vi "Text control 2 v6.3.vi"() -> ()   [LabVIEW 2016]
panel:
  in  "Tab Control":enum32{"Main", "Other parameters"}(tab)
  out "Line running":i32
  out "Total lines":i32
  out "Path":path=path "C:/users/rlp38/09Apr2009LTtesting/test2.txt"
  out "I vs Vg":cluster{"Y data in":dbl[], "X data in":dbl[]}[](graph)
  out "Is max":dbl format="%.2e"
  out "Id max":dbl format="%.2e"
  out "Ig max":dbl format="%.2e"
  out "Imax vs time":cluster{"Y data in":dbl[], "X data in":dbl[]}[](graph)
  out "Imin vs time":cluster{"Y data in":dbl[], "X data in":dbl[]}[](graph)
  out "I vs Vd":cluster{"Y data in":dbl[], "X data in":dbl[]}[](graph)
  in  "Script":string="#pulsedstressV d 0.03 20 0 0.5 0.0827 5\n#\n#itime m\n#gaterangemode a\n#drainrangemode a\n#pulsed on 0.05 0 0.02\n#transfer d -10 40 1 5 40 35\n#transfer d -10 40 1 5 40 35\n#transfer d -10 40 1 5 40 35\n#output d 0 40 20 0 40 1\n#\n#\n#sample 1 0.008 221 6 0.003\n#samplei 400e-6 200 6 0.002 0.1\n#vsu2pulse -10 4\n#\n#stressV 0.016 0.03 2e-4 0.1e-3 11\n#stressI 220e-7 0.08 15\n#transfer s -1 1 0.5 -0.005 0.005 0.005\n#output s 0 0 0 -0.008 0.008 0.002"
  out "Command running:":string
  out "Serial port data":string
  out "Elapsed Time":dbl caption="Elapsed Time (s)"
  in  "Time Units":u16(ring)=1 items=["Seconds", "Minutes", "Hours"]
  in  "Time Offset":dbl caption="Set Start Time (s)"
  in  "Reset":bool
  in  "Auto Reset":bool
  in  "integration time":u32(slide) max=2 step=1 scale=0.0..2.0
  out "Is on":dbl format="%.2e"
  out "Id on":dbl format="%.2e"
  out "Ig on":dbl format="%.2e"
  out "Ion vs time":cluster{"Y data in":dbl[], "X data in":dbl[]}[](graph)
  out "Ioff vs time":cluster{"Y data in":dbl[], "X data in":dbl[]}[](graph)
  out "Ig min":dbl format="%.2e"
  out "Id min":dbl format="%.2e"
  out "Is min":dbl format="%.2e"
  out "Is off":dbl format="%.2e"
  out "Id off":dbl format="%.2e"
  out "Ig off":dbl format="%.2e"
  in  "Integration time (long)":dbl=0.32 min=0.04 max=2.0 step=0.02 format="%.2f"
  in  "Integration time (short)":dbl=0.0019 min=8e-05 max=0.0019 step=8e-05 format="%^.0e"
  in  "Drain: Compliance":dbl=0.001 format="%.8f"
  in  "Gate: Compliance":dbl=0.001 format="%.8f"
  in  "Interrupt scan":bool
  in  "Standby":T1
  in  "Full Reset":bool
  in  "SMU4":cluster{"on/off":bool, "Voltage":dbl} {"Voltage" min=-100.0 max=100.0 format="%.2f"}
  in  "Interrupt program":bool
  in  "Gate Range\nmode":u16(ring) items=["Auto", "Limited", "Fixed"]
  in  "Gate Range":u8(slide)=6 max=11 scale=0.0..11.0
  in  "Source/Drain\nRange mode":u16(ring) items=["Auto", "Limited", "Fixed"]
  in  "Source/Drain Range":u8(slide)=6 max=11 scale=0.0..11.0
  in  "Panel Controls":T2={"Emergency Stop"=refnum, "TransGraph Max"=1e-05, "Text/Graph (text=false)"=TRUE} {"TransGraph Max" format="%.2e"}
  in  "Panel Controls 2":T3={"Emergency Stop"=refnum, "TransGraph Max"=1e-05, "Text/Graph (text=false)"=TRUE, "TransGraph Min"=1e-11} {"TransGraph Min" format="%.2e"; "TransGraph Max" format="%.2e"}
  out "error out":errorcluster
  in  "Delay before read (ms)":u32=1000
  in  "byte count":u32=64
  in  "Serial End Mode for Reads":u16(ring)=2 items=["None", "LastBit", "TermChar"]
  in  "Timeout (ms)":u32=10000
  in  "Enable Termination\nChar (T)":bool=TRUE
  in  "Termination char\n(0xA = '\\n' = LF)\n(0xD = '\\r' = CR)":u8=13 format="%.0x"
  in  "flow control":u16(ring) items=["None"=0, "XON/XOFF"=1, "RTS/CTS"=2, "DTR/DSR"=4]
  in  "stop bits":u16(ring)=10 items=["1.0"=10, "1.5"=15, "2.0"=20]
  in  "parity":u16(ring) items=["None", "Odd", "Even", "Mark", "Space"]
  in  "data bits":u16=8 min=5 max=8 step=1
  in  "VISA resource name":refnum<visa-resource-name>="COM6"
  in  "baud rate":u32=9600
  out "Timings Indicator":T4
  in  "Timings (overwritten by the Front Panel)":T5={"integration time"=0, "Short/Long integration time"=0.00064, "hold time (sec)"=0.0, "delay time (sec)"=0.0, "Step Time (0 disables)"=0.0, "sweep method"=0, "Pulse period"=0.005, "Base voltage"=0.0, "Pulse width"=0.0005} {"Pulse width" min=0.0005 max=0.1 step=0.0001 format="%.4f"; "Base voltage" format="%^.4e"; "Pulse period" min=0.005 max=1.0 step=0.0001 format="%.4f"; "sweep method" items=["Continuous", "Pulsed"]; "Step Time (0 disables)" format="%.2f"; "delay time (sec)" format="%.4f"; "hold time (sec)" format="%.4f"; "Short/Long integration time" format="%^.0e"; "integration time" scale=0.0..2.0}
  in  "Gate":T6={"Gate Start"=0.0, "Gate Stop"=2.0, "Gate Step (linear only)"=1.0, "Gate Compliance"=0.0001, "Gate PComp"=0.0, "Range mode"=0, "Range"=6} {"Range" max=11 scale=0.0..11.0; "Range mode" items=["Auto", "Limited", "Fixed"]; "Gate PComp" format="%^.2e"; "Gate Compliance" format="%^.2e"; "Gate Step (linear only)" format="%^.4e"; "Gate Stop" format="%^.4e"; "Gate Start" format="%^.4e"}
  in  "Drain 2":T7={"Drain Start"=0.0, "Drain Stop"=2.0, "Drain Compliance"=0.0001, "Drain Step"=1.0, "Drain PComp"=0.0, "Range mode"=0, "Range"=6} {"Range" max=11 scale=0.0..11.0; "Range mode" items=["Auto", "Limited", "Fixed"]; "Drain PComp" format="%^.2e"; "Drain Step" format="%^.4e"; "Drain Compliance" format="%^.2e"; "Drain Stop" format="%^.4e"; "Drain Start" format="%^.4e"}
  # "Time"
  # "Syntax:\nitime [s|m|l] time(sec): [s|m|l] determines the integration time setting (small|medium|long) and time sets the value.\nNOTE: The value of the integration time has to be within the range allowed by its category (s|m|l), otherwise, the closest value will be used. (e.g. if the category is set to short but the time value is very long, the actual value used will be the maximum short integration time.\nIntegration times:\n    Short: Default: 640 us. Range: 8E-5 - 1.92E-3 seconds.\n    Medium: Fixed at 1 NPL cycle (0.02 seconds).\n    Long: Default: 16 NPL cycles (0.32 seconds). Range: 2-100 NPL cycles (0.04 seconds - 2 seconds).\ngaterangemode [a|l|f]\ndrainrangemode [a|l|f]\npulsed [on|off] PulsePeriod(sec) PulseBaseVoltage PulseONWidth(sec)\nstandby [on l off]\nwait NumMilliseconds\nwait-min NumMinutes\n# texthere = comment\ntransfer [s|d] VgStart VgStop VgStep VdStart VdStop VdStep\noutput [s|d] VgStart VgStop VgStep VdStart VdStop VdStep\nsample Vg Vd NumSamples Time(s) SampleInterval(s)\nsamplei Idg NumSamples Time(s) SampleInterval(s) VDGcompliance\n100 samples is approximately 13 seconds with medium integration\n# if in doubt use SampleInterval(s) = 0.004\nstressV VG VD IGcompliance IDcompliance Duration(sec)\nstressI IDG VDGcompliance Duration(sec)\nvsu2pulse Bias Duration(s)\npulsedstressV [s|d] VEstop VgON VgOFF Period(s) PulseONwidth(s) Vd\nsample-fpp Vg Vd NumSamples Time\nresample-fpp Vg Vd\ntransfer-fpp [s|d] VgStart VgStop VgStep VdStart VdStop VdStep\noutput-fpp [s|d] VgStart VgStop VgStep VdStart VdStop VdStep\nserial SerialPortCommand"
  # "1\n2\n3\n4\n5\n6\n7\n8\n9\n10\n11\n12\n13\n14\n15\n16\n17\n18\n19\n20"
  # "Serial port settings"
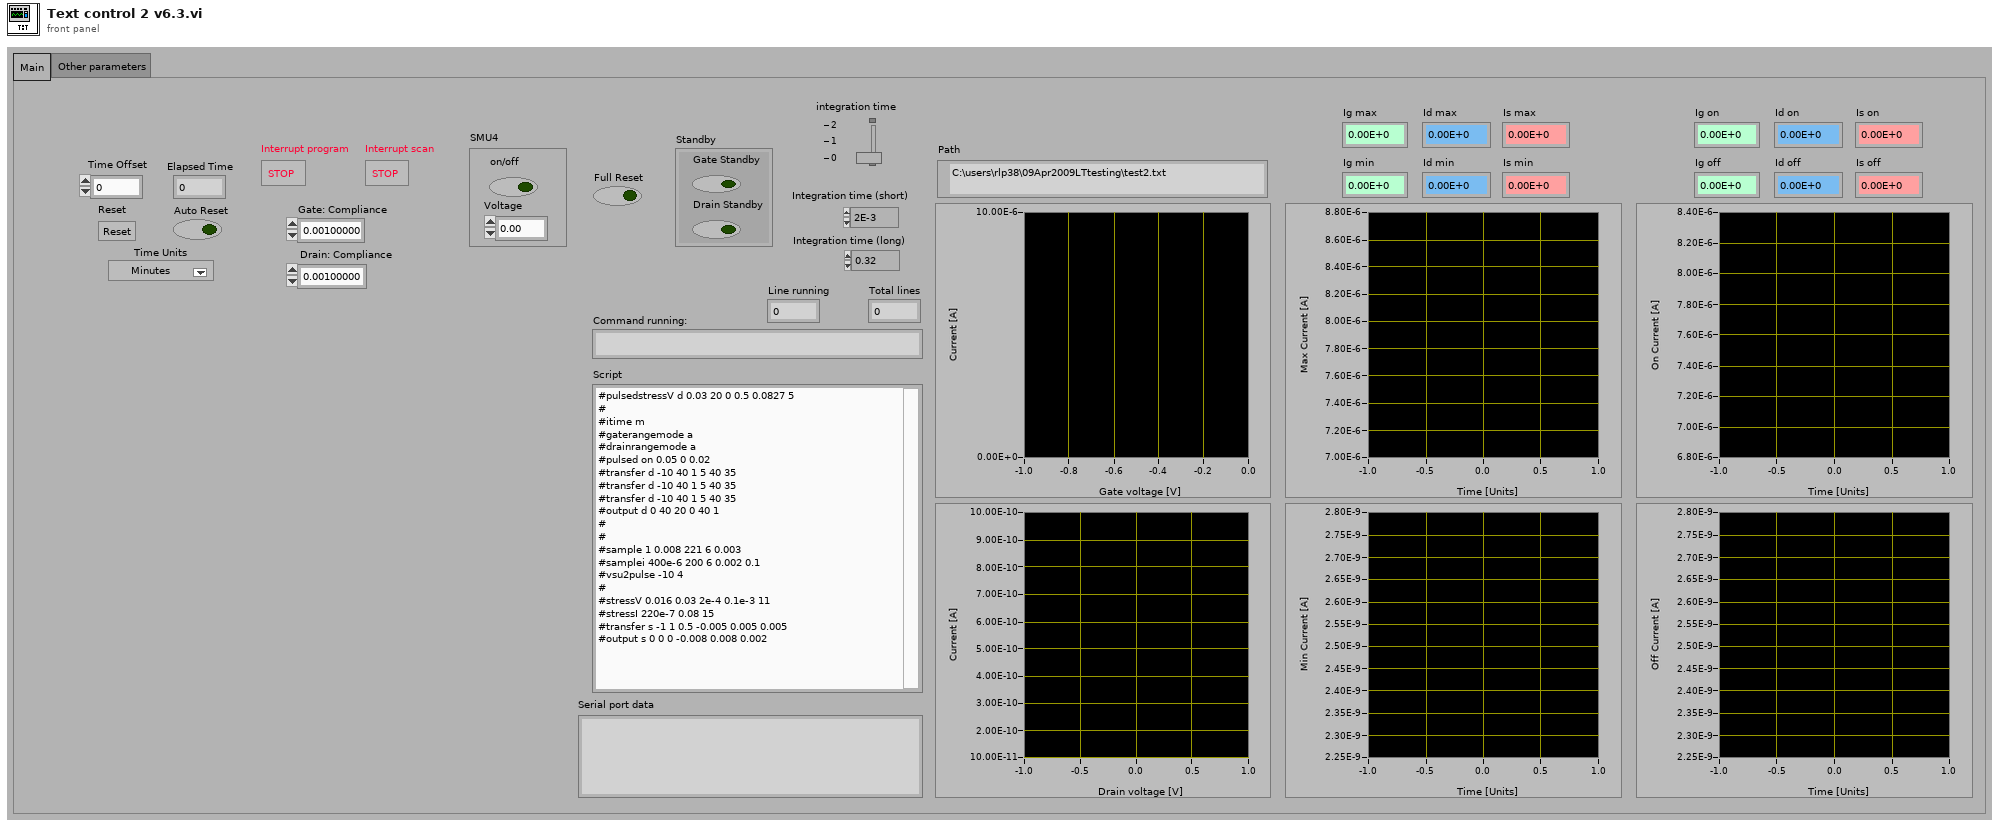
[diagram p1: front panel]
types:
  T1 = cluster{"Gate Standby":bool, "Drain Standby":bool}
  T2 = cluster{"Emergency Stop":refnum<vi>, "TransGraph Max":dbl, "Text/Graph (text=false)":bool}
  T3 = cluster{"Emergency Stop":refnum<vi>, "TransGraph Max":dbl, "Text/Graph (text=false)":bool, "TransGraph Min":dbl}
  T4 = cluster{"integration time (0:s, 1:m, 2:l)":u32, "Short/Long integration time":dbl, "hold time (sec)":dbl, "delay time (sec)":dbl, "Step Time (0 disables)":dbl, "sweep method":u16, "Pulse period":dbl, "Base voltage":dbl, "Pulse width":dbl}
  T5 = cluster{"integration time":u32, "Short/Long integration time":dbl, "hold time (sec)":dbl, "delay time (sec)":dbl, "Step Time (0 disables)":dbl, "sweep method":u16, "Pulse period":dbl, "Base voltage":dbl, "Pulse width":dbl}
  T6 = cluster{"Gate Start":dbl, "Gate Stop":dbl, "Gate Step (linear only)":dbl, "Gate Compliance":dbl, "Gate PComp":dbl, "Range mode":u16, "Range":u8}
  T7 = cluster{"Drain Start":dbl, "Drain Stop":dbl, "Drain Compliance":dbl, "Drain Step":dbl, "Drain PComp":dbl, "Range mode":u16, "Range":u8}
  T8 = enum16{"open", "replace", "create", "open or create", "replace or create", "replace or create with confirmation"}
  T9 = cluster{"V2 Start":dbl, "V2 Step":dbl, "Number of points":i32}
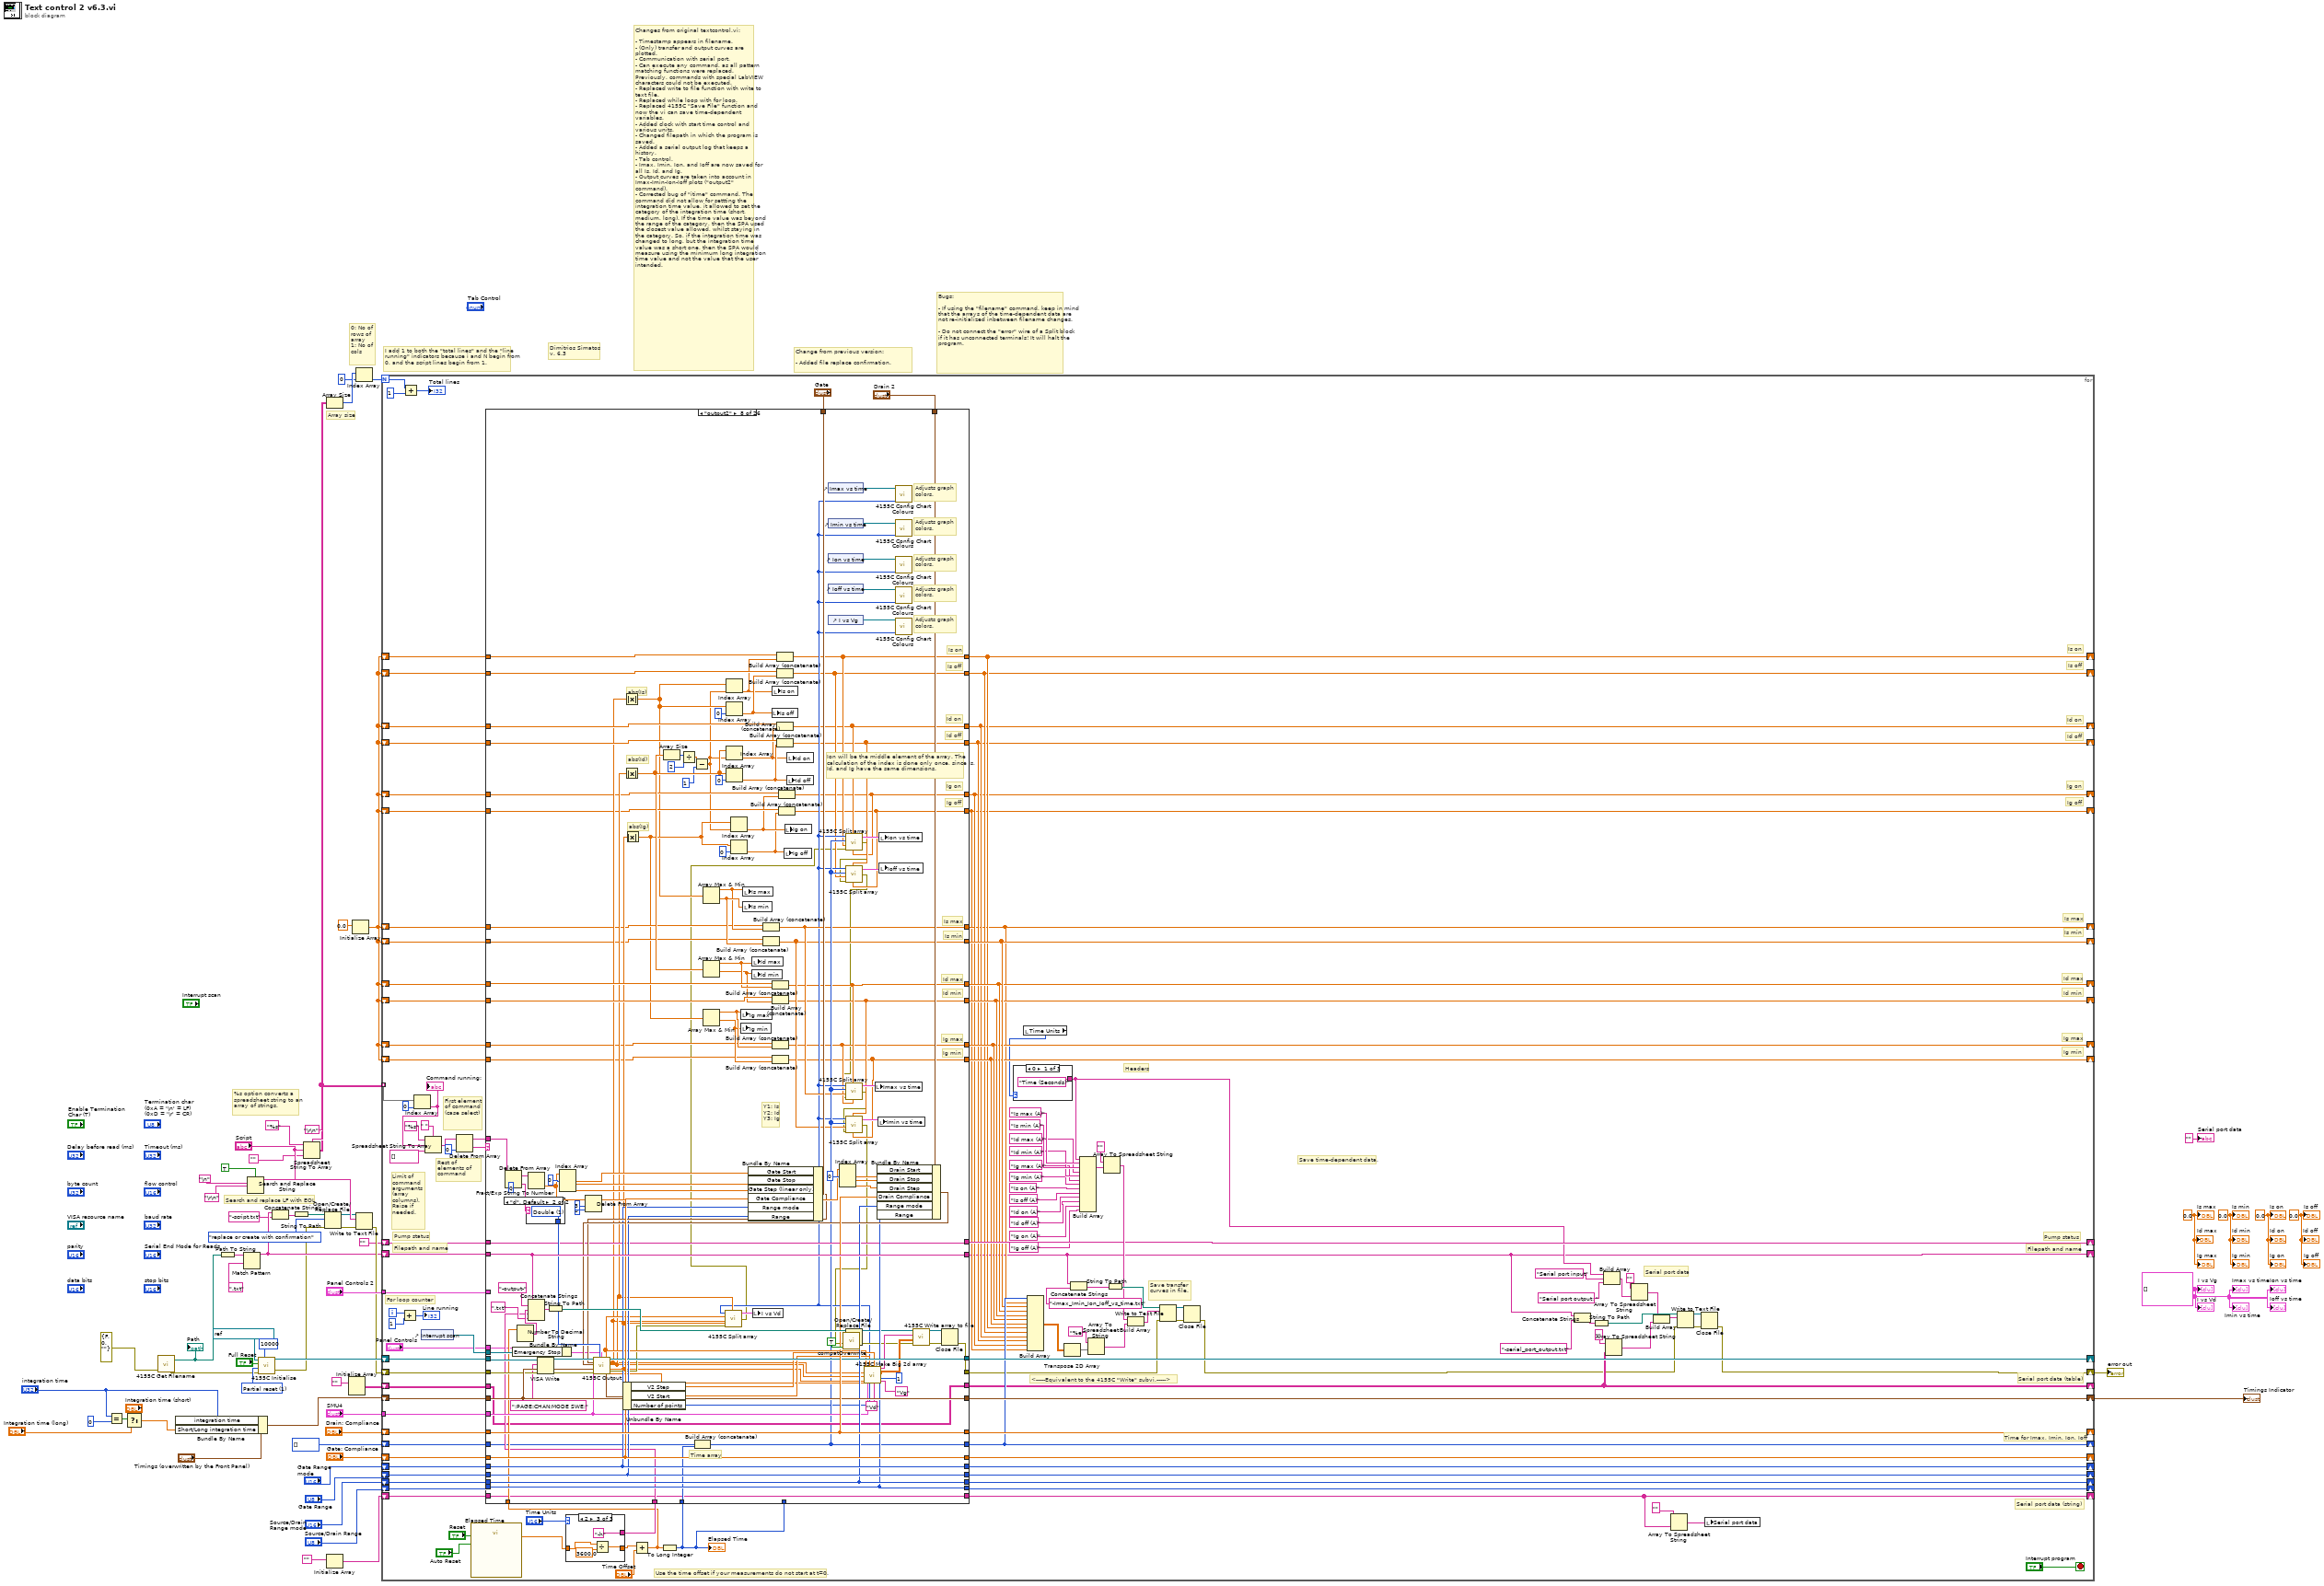
[diagram p0: block diagram]
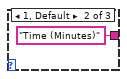
[diagram p2: hidden frame]
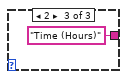
[diagram p3: hidden frame]
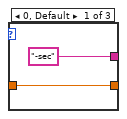
[diagram p4: hidden frame]
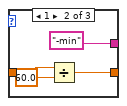
[diagram p5: hidden frame]
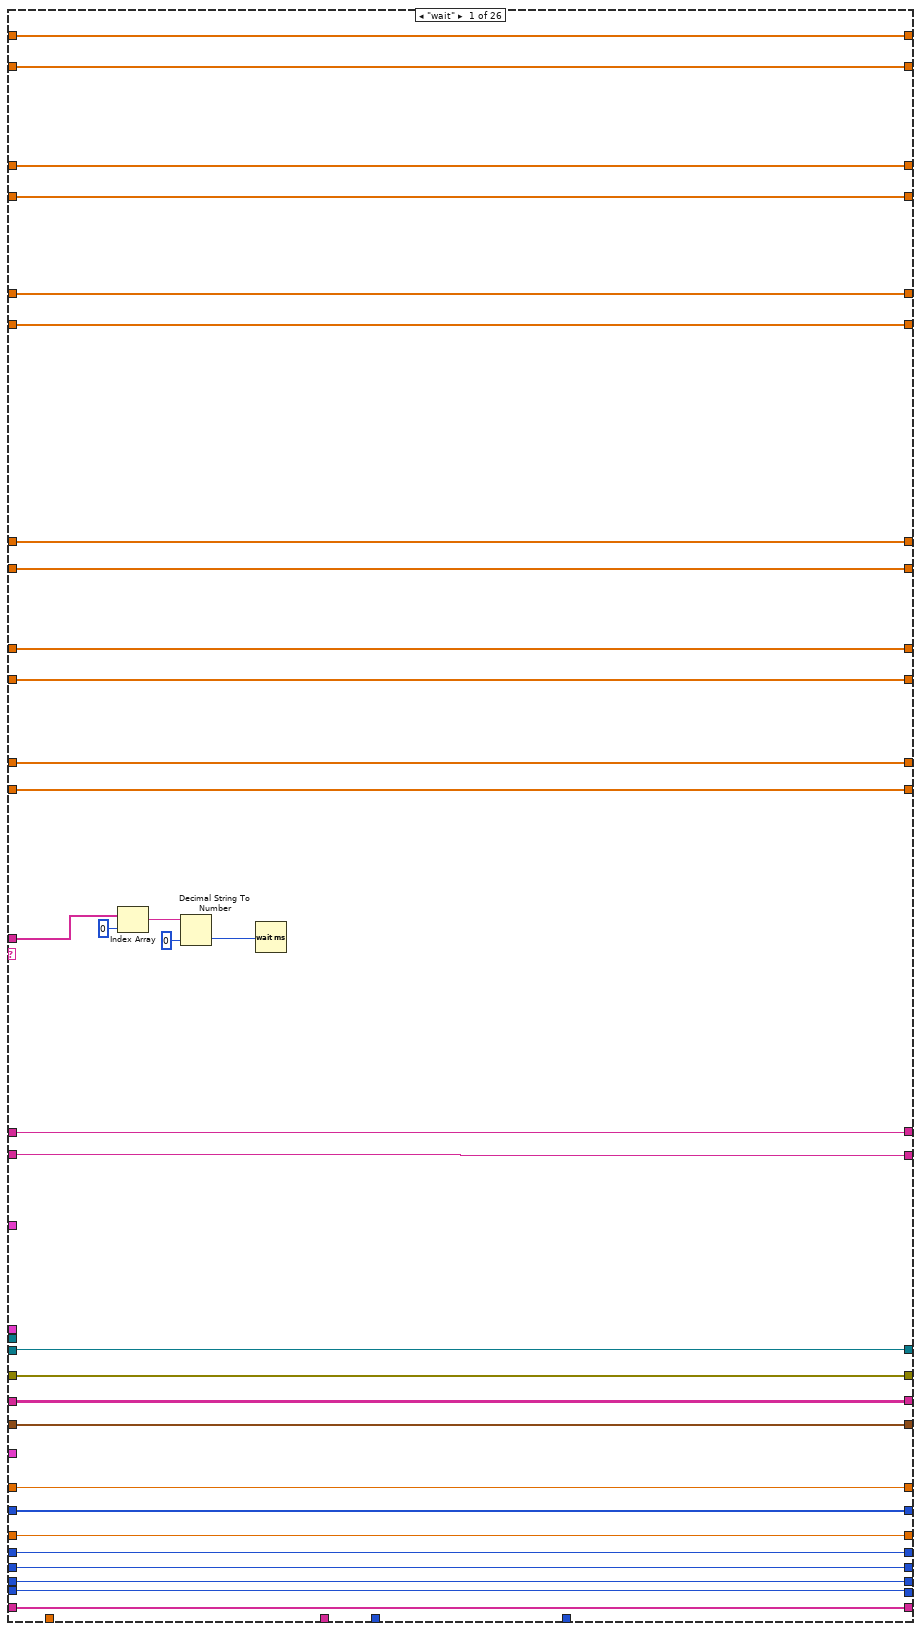
[diagram p6: hidden frame]
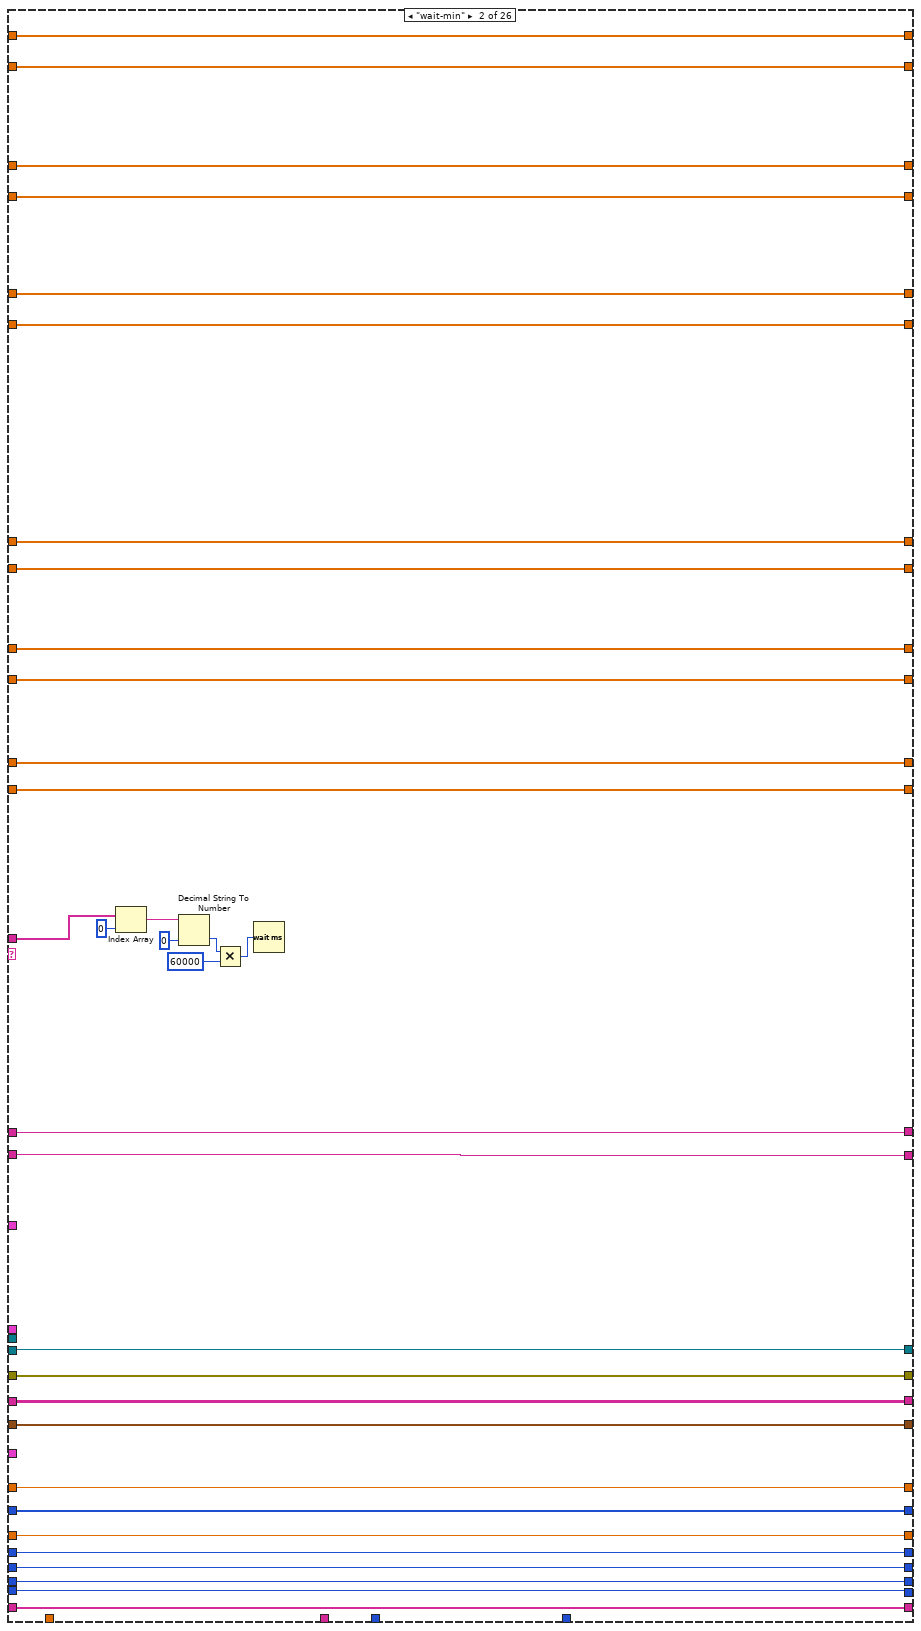
[diagram p7: hidden frame]
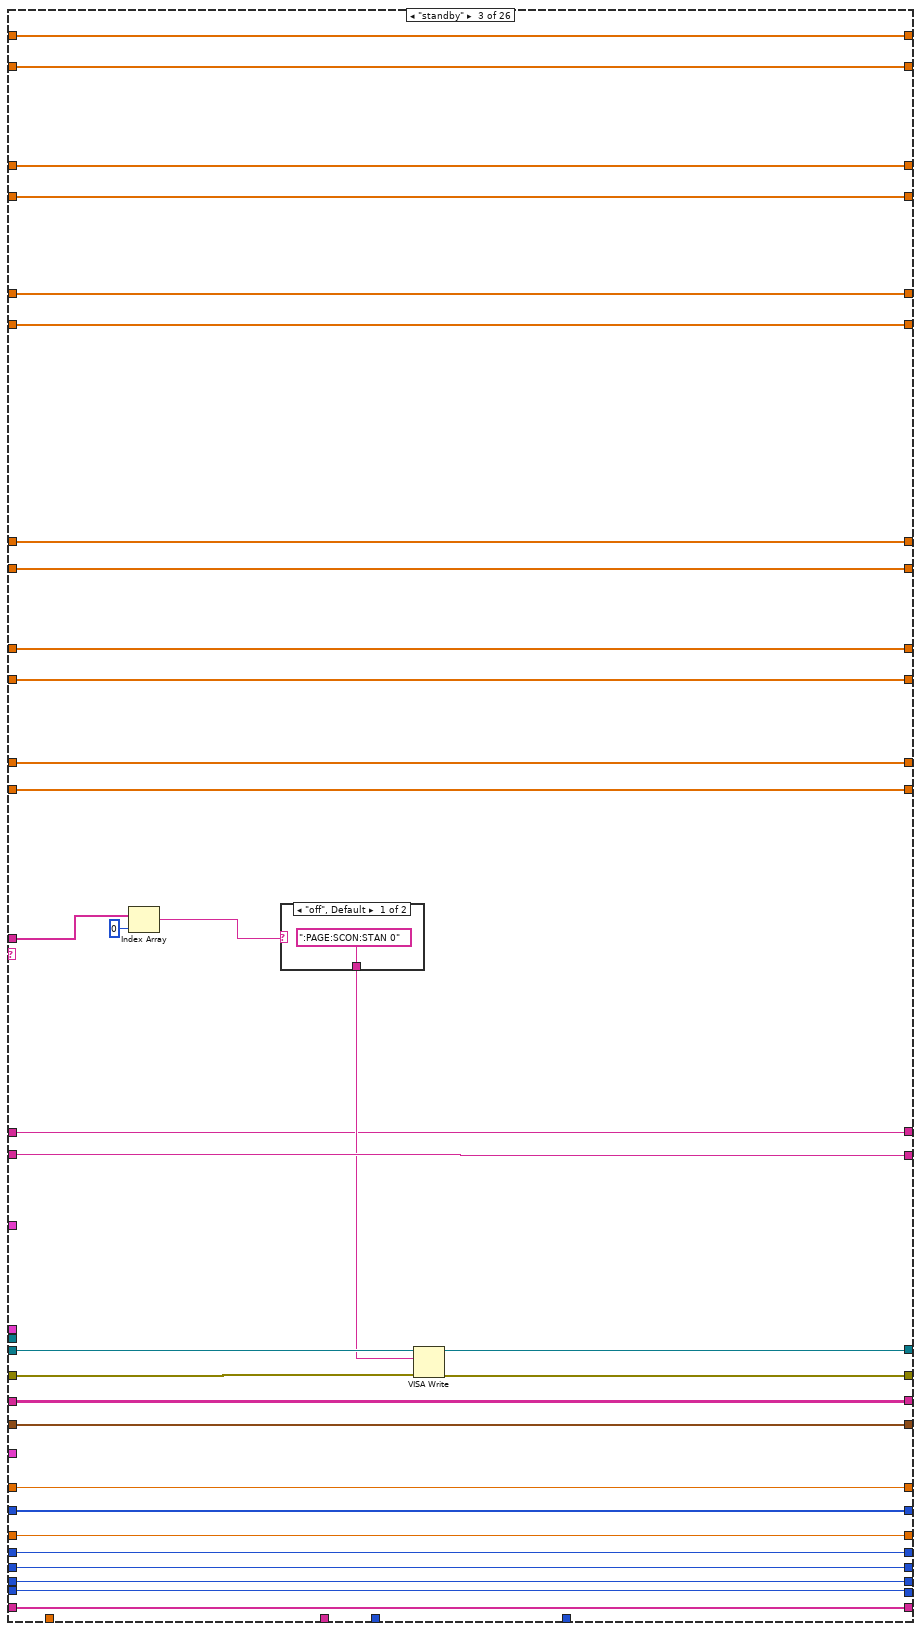
[diagram p8: hidden frame]
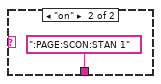
[diagram p9: hidden frame]
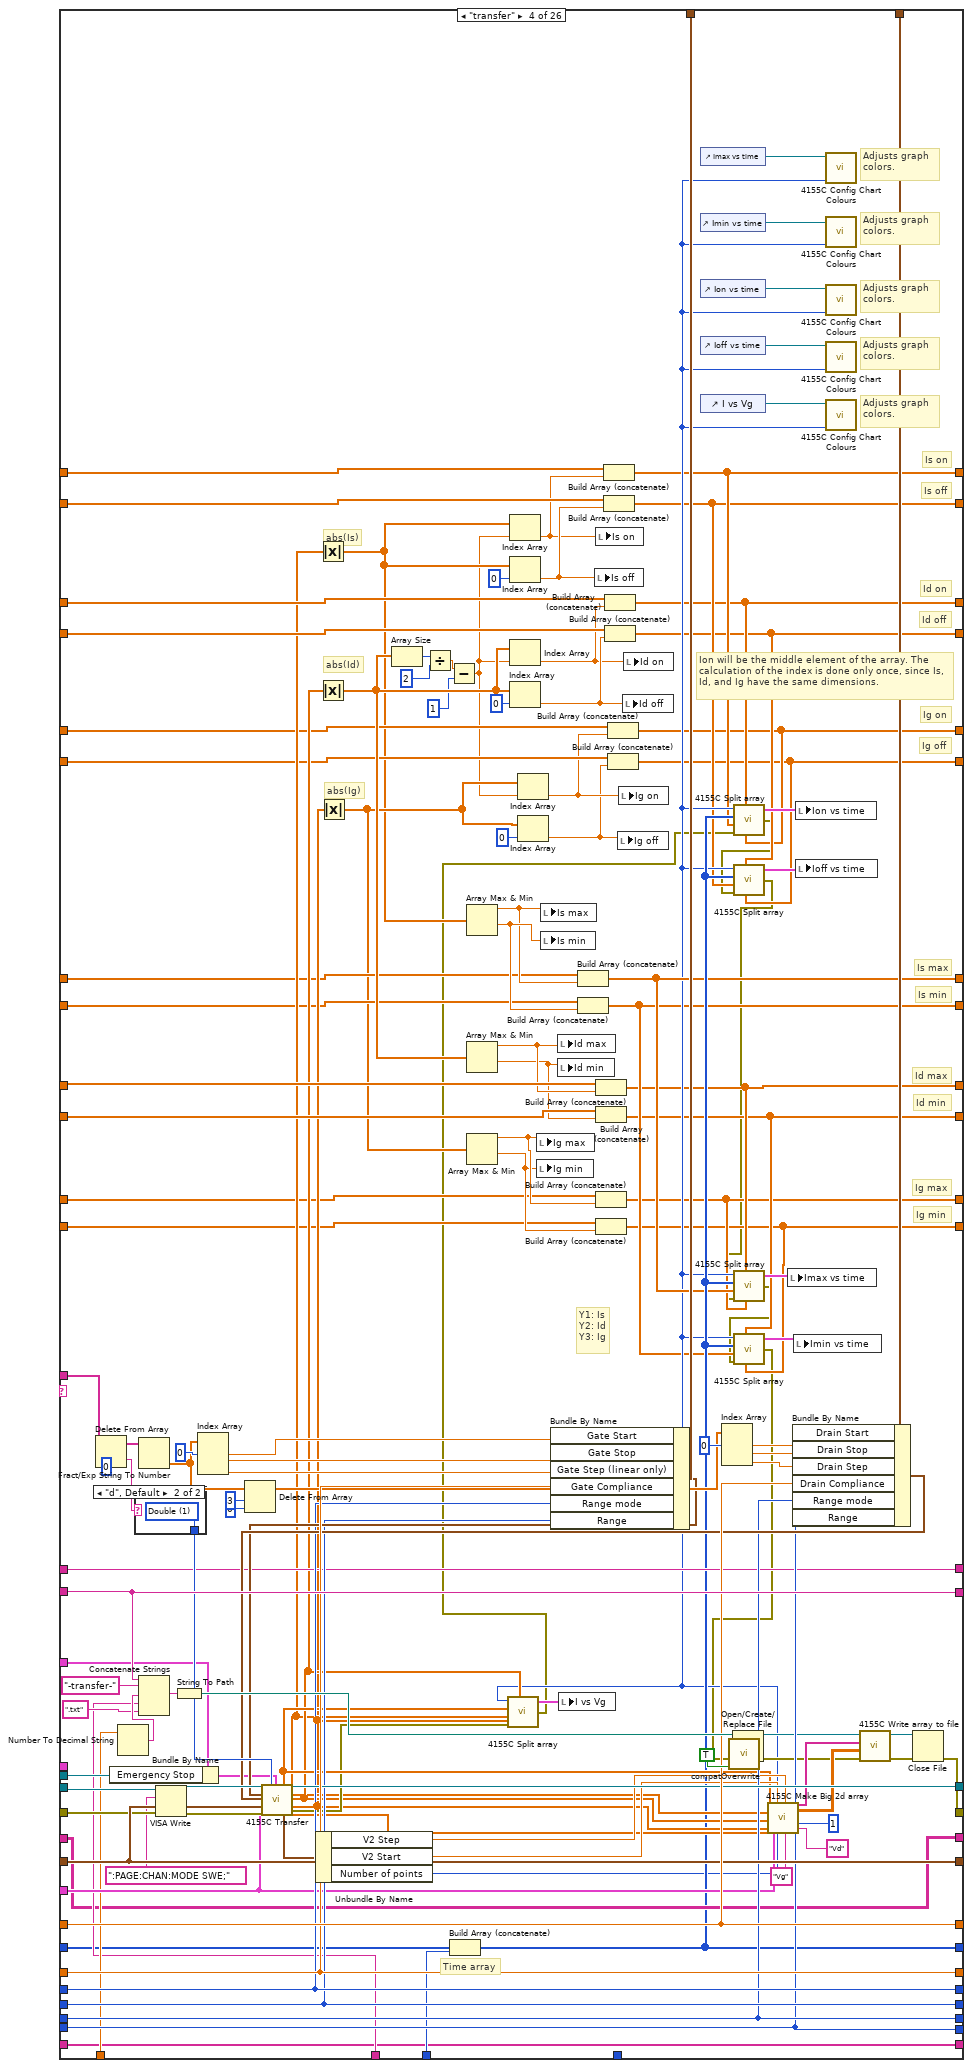
[diagram p10: hidden frame]
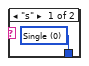
[diagram p11: hidden frame]
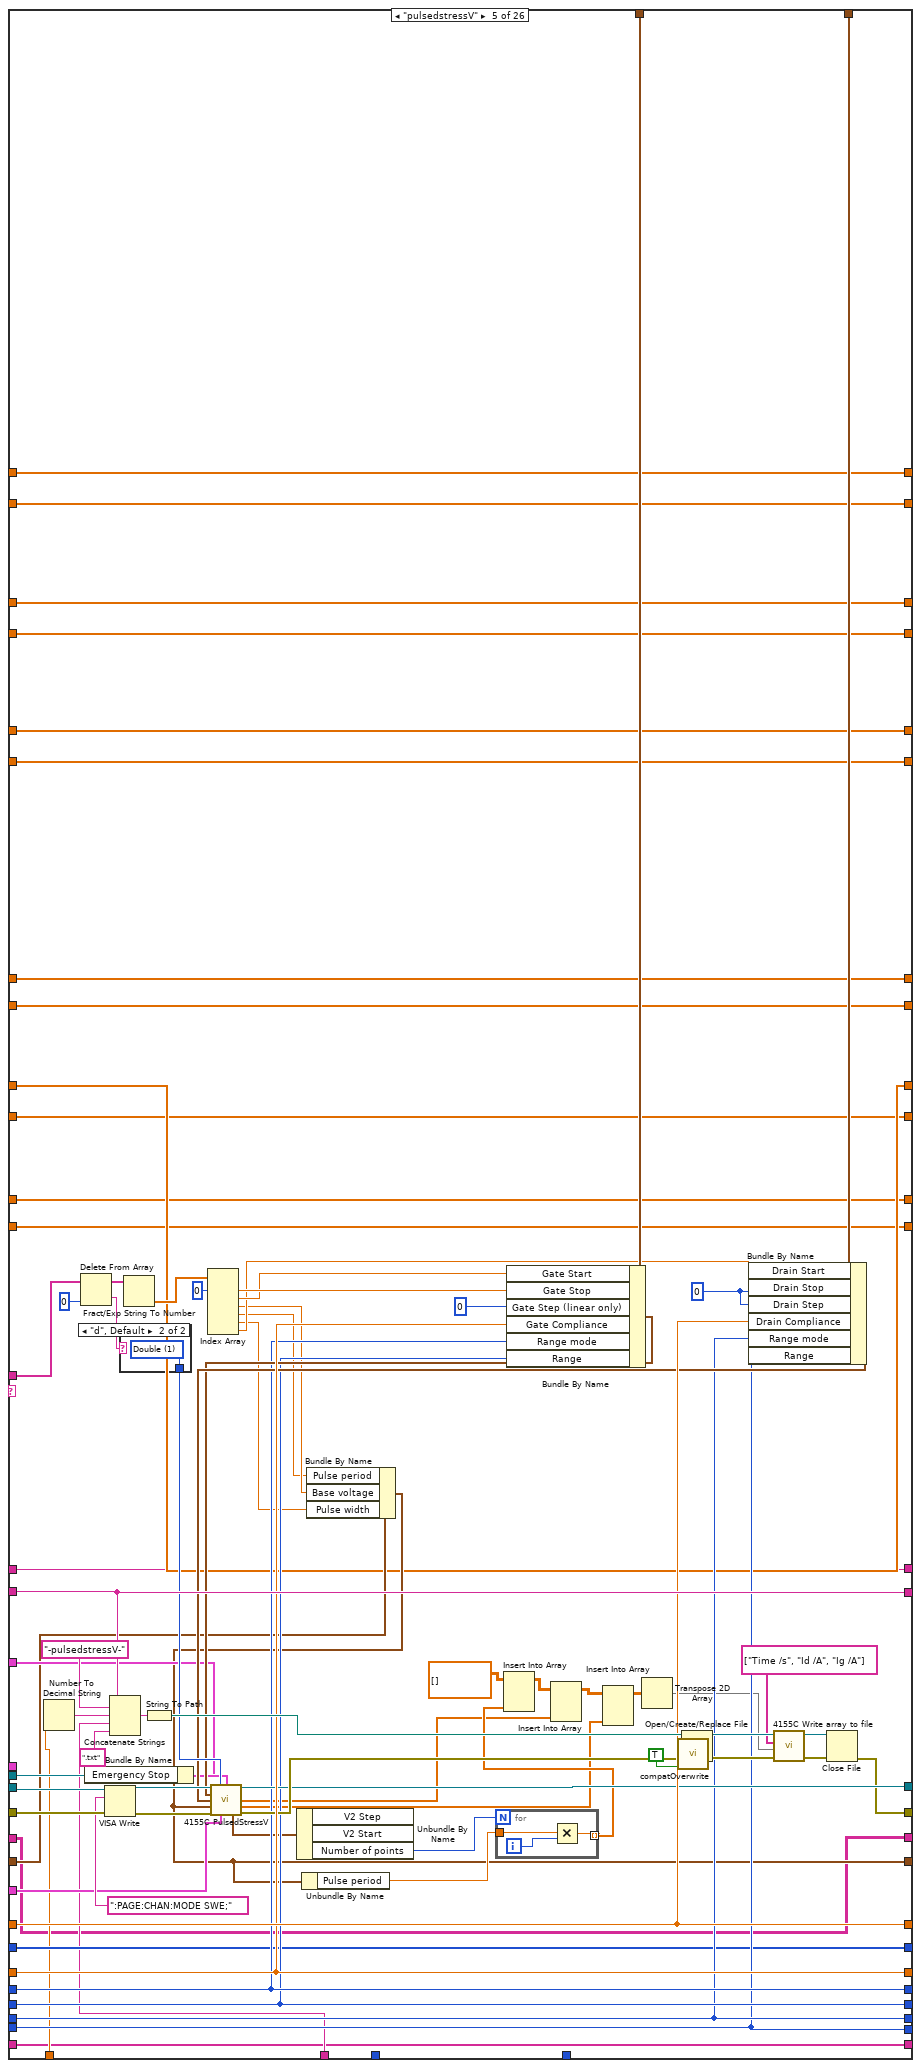
[diagram p12: hidden frame]
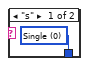
[diagram p13: hidden frame]
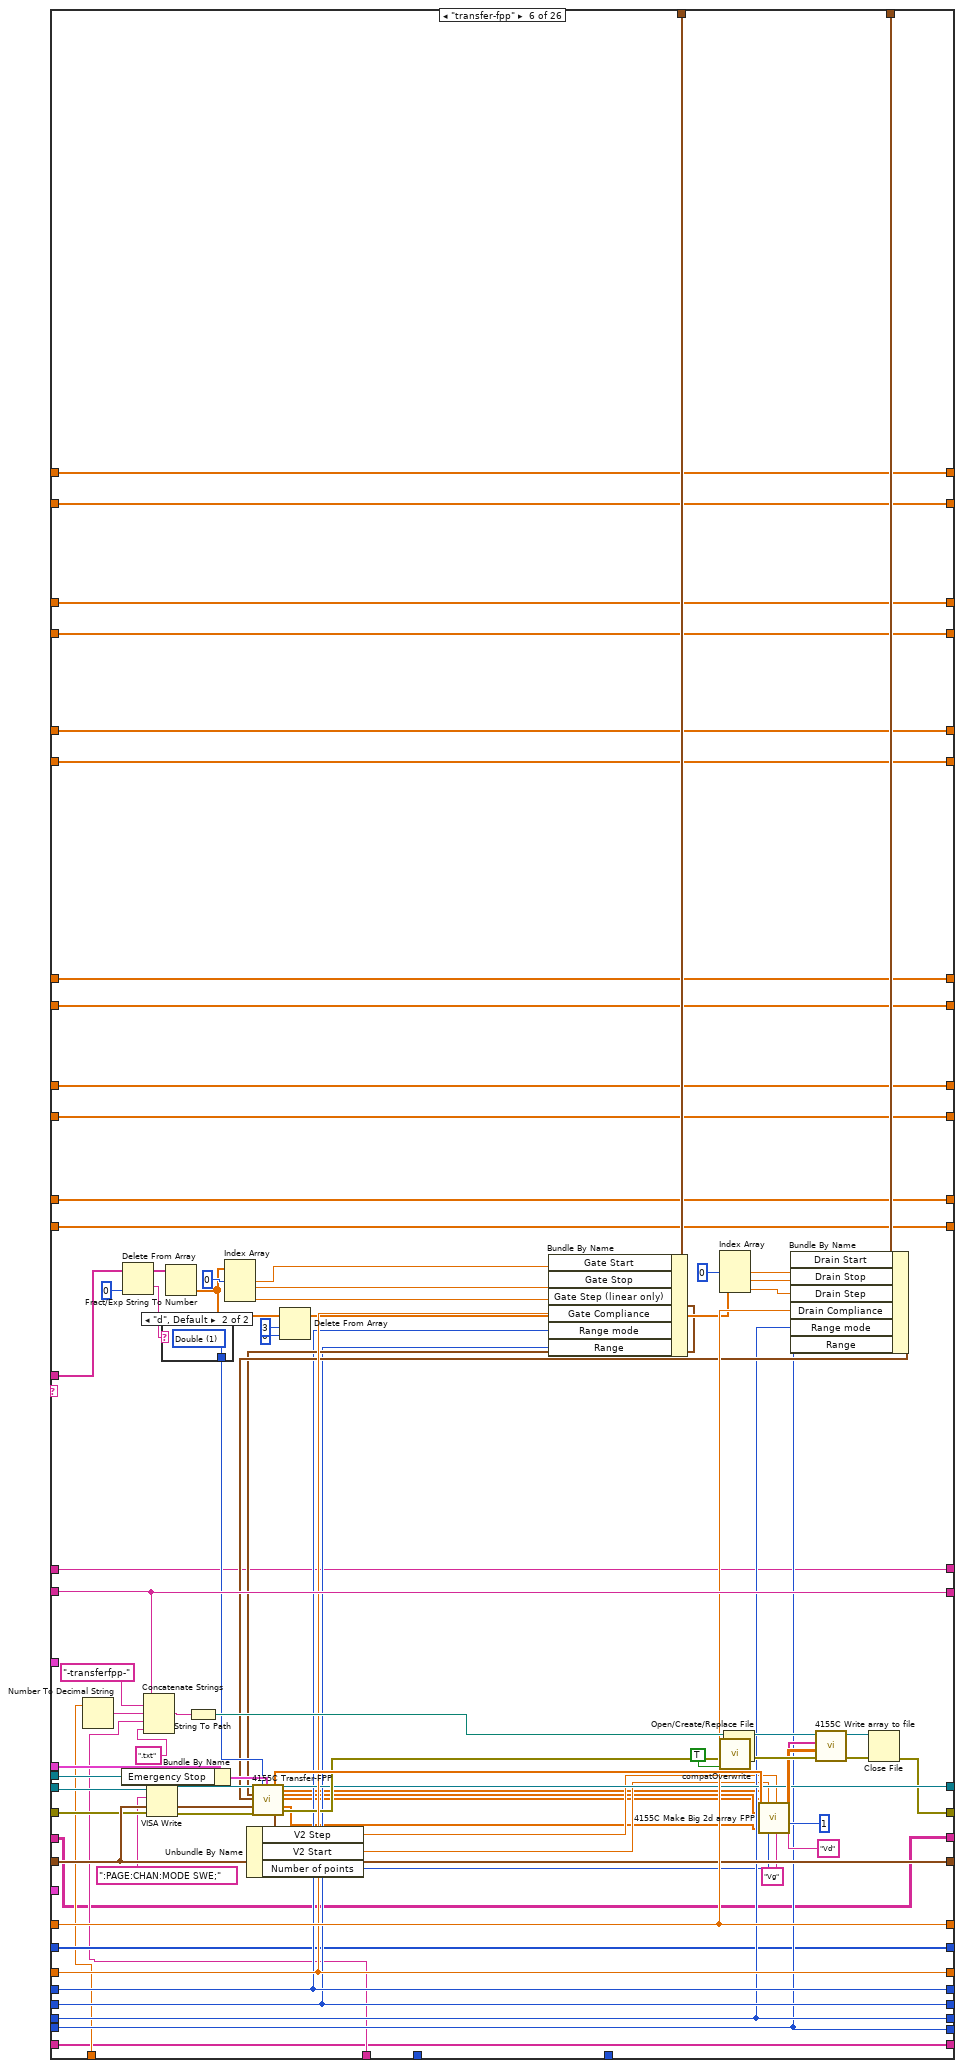
[diagram p14: hidden frame]
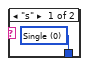
[diagram p15: hidden frame]
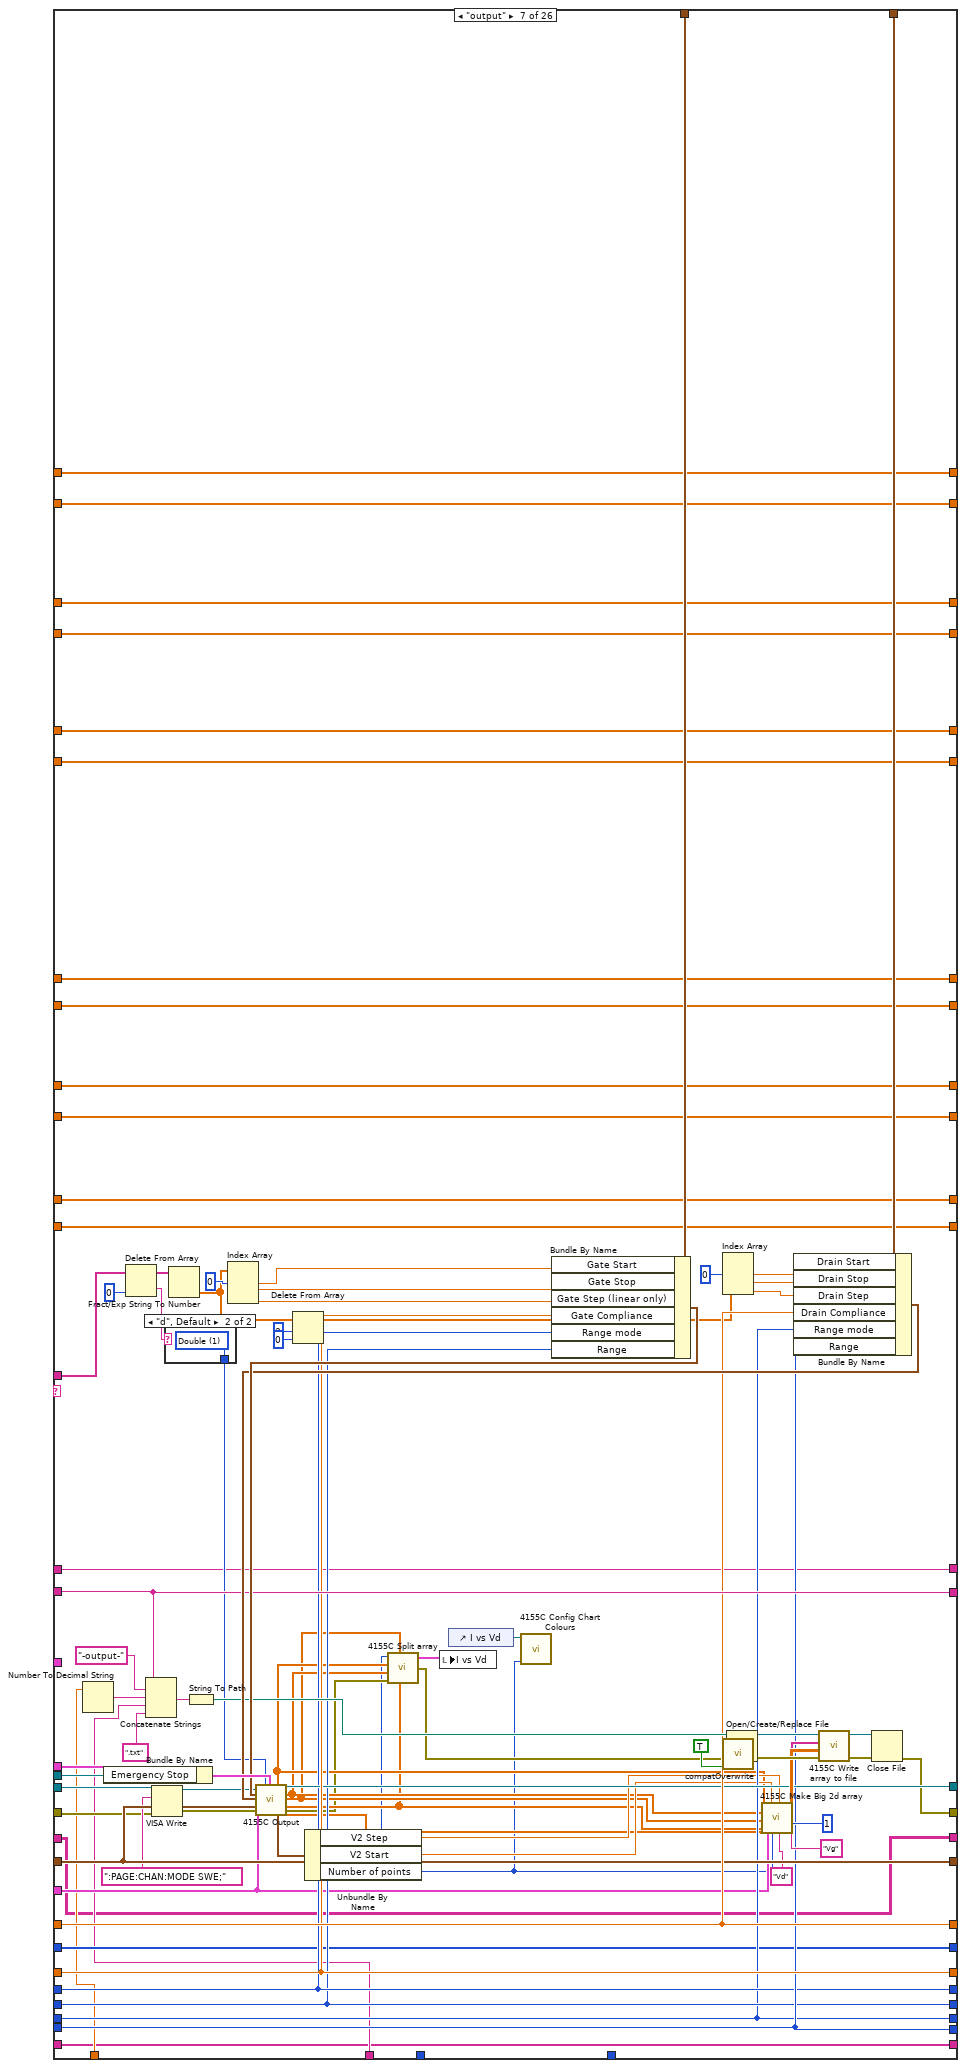
[diagram p16: hidden frame]
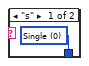
[diagram p17: hidden frame]
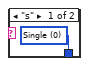
[diagram p18: hidden frame]
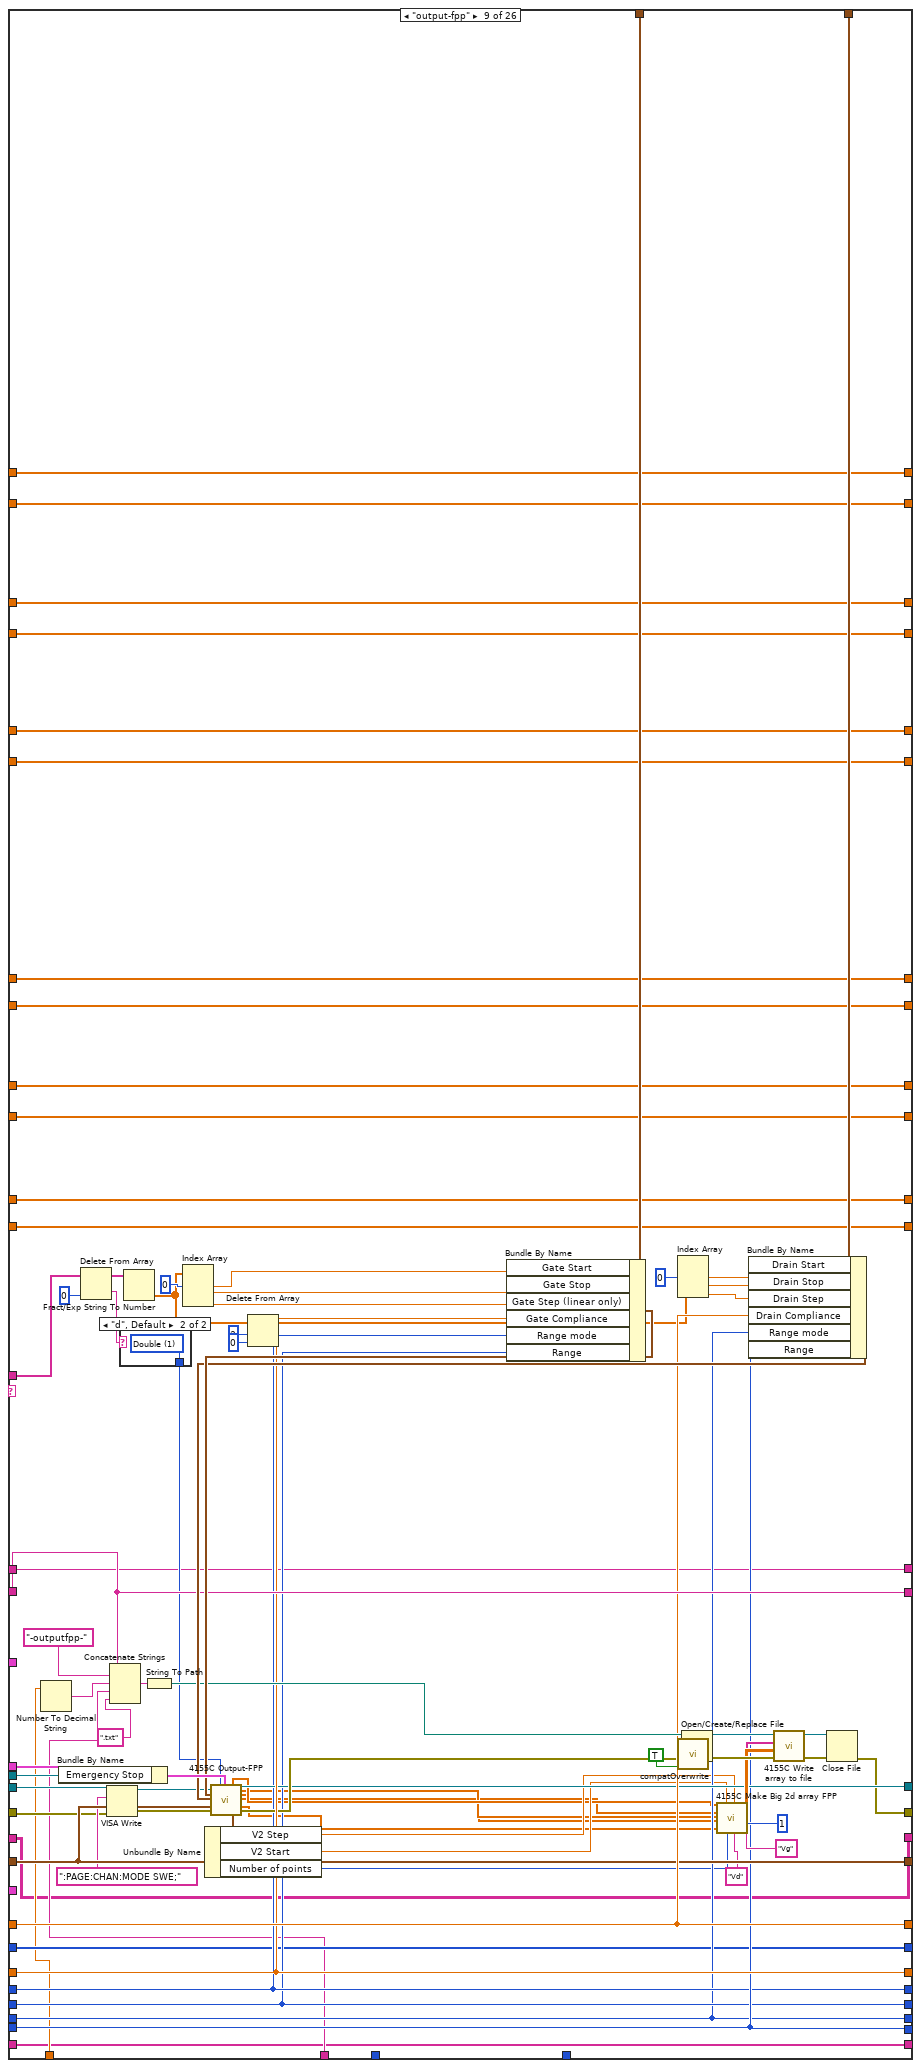
[diagram p19: hidden frame]
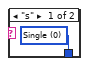
[diagram p20: hidden frame]
diagram:
  w7 = cluster{"Y data in":dbl[], "X data in":dbl[]}[] [] ("I vs Vg")
  w8 = 0.0 ("Is off")
  w9 = 0.0 ("Is on")
  w10 = 0.0 ("Is min")
  w11 = 0.0 ("Is max")
  w58 = u16 1 items=["Reset All", "Partial reset"] ("Type of reset")
  # "Change from previous version:\n\n- Added file replace confirmation."
  # "I add 1 to both the \"total lines\" and the \"line running\" indicators because i and N begin from 0, and the script lines begin from 1."
  # "Bugs:\n\n- If using the \"filename\" command, keep in mind that the arrays of the time-dependent data are not re-initialized inbetween filename changes. \n\n- Do not connect the \"error\" wire of a Split block if it has unconnected terminals! It will halt the program."
  # "Array size"
  # "%s option converts a spreadsheet string to an array of strings."
  # "0: No of rows of array\n1: No of cols"
  # "Dimitrios Simatos\nv. 6.3"
  # "Changes from original textcontrol.vi:\n\n- Timestamp appears in filename.\n- (Only) transfer and output curves are plotted.\n- Communication with serial port.\n- Can execute any command, as all pattern matching functions were replaced. Previously, commands with special LabVIEW characters could not be executed.\n- Replaced write to file function with write to text file.\n- Replaced while loop with for loop.\n- Replaced 4155C \"Save File\" function and now the vi can save time-dependent variables.\n- Added clock with start time control and various units.\n- Changed filepath in which the program is saved.\n- Added a serial output log that keeps a history.\n- Tab control.\n- Imax, Imin, Ion, and Ioff are now saved for all Is, Id, and Ig.\n- Output curves are taken into account in Imax-Imin-Ion-Ioff plots (\"output2\" command).\n- Corrected bug of \"itime\" command. The command did not allow for settting the integration time value, it allowed to set the category of the integration time (short, medium, long). If the time value was beyond the range of the category, then the SPA used the closest value allowed, whilst staying in the category. So, if the integration time was changed to long, but the integration time value was a short one, then the SPA would measure using the minimum long integration time value and not the value that the user intended."
  # "Search and replace LF with EOL"
  n1 = Equal?(x="integration time", y=u32 0) -> (x = y?=w59:bool)
  n2 = Select(t="Integration time (short)", s=w59, f="Integration time (long)") -> (s? t:f=w16:dbl)
  n3 = call "4155C Get Filename.vi"("error in (no error)"=errorcluster {"status"=FALSE, "code"=0, "source"=""}) -> ("error out"=w53:errorcluster, "path"=w28:path)  [unwired: 2 in, 1 out]
  "Path" <- w28
  n4 = Bundle By Name(cluster="Timings (overwritten by the Front Panel)", "integration time"="integration time", "Short/Long integration time"=w16) -> (w51:T5)
  n5 = Path To String(path=w28) -> (string=w29:string)
  n6 = Match Pattern(string=w29, regular expression=".txt") -> (before substring=w14:string)  [unwired: 1 in, 3 out]
  n7 = Search and Replace String(replace all?=TRUE ("replace all? (F)"), input string="Script", search string="\n", replace string="\r\n") -> (result string=w41:string)  [unwired: 4 in, 3 out]
  n8 = call "4155C Initialise.vi"("VISA resource name in"=refnum<visa-resource-name> "GPIB0::14::INSTR", "Reset"="Full Reset", "Type of reset"=w58, "error in (no error)"=w53, "VISA Timeout Value"=u32 10000) -> ("VISA Resource Name out"=w52:refnum<visa-resource-name>, "error out"=w5:errorcluster)
  n9 = Concatenate Strings(w14, "-script.txt" ("string")) -> (w15:string)
  n10 = String To Path(string=w15) -> (path=w3:path)
  n11 = Spreadsheet String To Array(delimiter (Tab)="\r\n", format string="%s", spreadsheet string="Script", array type (2D Dbl)="") -> (array=w32:string[][])
  n12 = Open/Create/Replace File(file path (use dialog)=w3, error in=w5, operation (0:open)=T8."replace or create with confirmation") -> (refnum out=w2:refnum<file>, error out=w4:errorcluster)  [unwired: 3 in, 1 out]
  n13 = Array Size(array=w32) -> (size(s)=w36:i32[])
  n14 = Initialize Array("") -> (w21:string[])  [unwired: 1 in]
  n15 = Initialize Array("") -> (w19:string[][])  [unwired: 2 in]
  n16 = Initialize Array(0.0 ("element")) -> (w23:dbl[])  [unwired: 1 in]
  n17 = Index Array(array=w36, index=0) -> (element=w34:i32)
  n18 = Write to Text File(file (use dialog)=w2, text=w41, error in=w4) -> (error out=w25:errorcluster)  [unwired: 1 in, 2 out]
  n19 = for {
    N: w34 -> [w133]
    tunnel: "SMU4" -> [w169]
    shift-left: "Source/Drain Range" -> [w174]
    shift-right: [w170] -> _
    shift-left: "Source/Drain\nRange mode" -> [w175]
    shift-right: [w171] -> _
    shift-left: "Gate Range" -> [w176]
    shift-right: [w172] -> _
    shift-left: "Gate Range\nmode" -> [w177]
    shift-right: [w173] -> _
    shift-left: "Gate: Compliance" -> [w186]
    shift-right: [w182] -> _
    shift-left: "Drain: Compliance" -> [w187]
    shift-right: [w183] -> _
    shift-left: w51 -> [w188]
    shift-right: [w184] -> w17
    shift-left: w25 -> [w189]
    shift-right: [w67] -> w27
    shift-left: w52 -> [w190]
    shift-right: [w185] -> _
    shift-left: w14 -> [w191]
    shift-right: [w70] -> _
    tunnel: "Panel Controls 2" -> [w168]
    shift-right: [w82] -> _
    shift-left: w23 -> [w167]
    shift-right: [w118] -> _
    shift-left: i32[] [] -> [w163]
    tunnel: w32 -> [w162] mode=indexing
    shift-right: [w81] -> _
    shift-left: w23 -> [w139]
    shift-right: [w112] -> _
    shift-left: w21 -> [w125]
    shift-right: [w120] -> _
    shift-left: "" -> [w119]
    shift-right: [w113] -> _
    shift-left: w19 -> [w115]
    shift-right: [w75] -> _
    shift-left: w23 -> [w103]
    shift-right: [w76] -> _
    shift-left: w23 -> [w102]
    shift-right: [w80] -> _
    shift-left: w23 -> [w91]
    shift-right: [w79] -> _
    shift-left: w23 -> [w90]
    shift-right: [w73] -> _
    shift-left: w23 -> [w89]
    shift-right: [w83] -> _
    shift-left: w23 -> [w88]
    shift-right: [w74] -> _
    shift-left: w23 -> [w87]
    shift-right: [w72] -> _
    shift-left: w23 -> [w86]
    shift-right: [w78] -> _
    shift-left: w23 -> [w85]
    shift-right: [w77] -> _
    shift-left: w23 -> [w84]
    i -> [w128]
    stop <- "Interrupt program" stop-if-true
    # "Is off"
    # "Is on"
    # "Ig off"
    # "Ig on"
    # "Is min"
    # "Is max"
    # "Ig min"
    # "Ig max"
    # "Id min"
    # "Id max"
    # "Id off"
    # "Id on"
    # "Pump status"
    # "Filepath and name"
    # "Pump status"
    # "Limit of command arguments (array columns). Raise if needed."
    # "Serial port data (string)"
    # "Serial port data (table)"
    # "Serial port data"
    # "For loop counter"
    # "<-----Equivalent to the 4155C \"Write\" subvi.----->"
    # "Headers"
    # "Save transfer curves in file."
    # "Filepath and name"
    # "Save time-dependent data."
    # "Use the time offset if your measurements do not start at t=0."
    # "Time for Imax, Imin, Ion, Ioff"
    # "Rest of elements of command"
    # "First element of command\n(case select)"
    n20 = Add(x=w128, y=1) -> (x+y=→"Line running":i32)
    n21 = Add(x=w133, y=1) -> (x+y=→"Total lines":i32)
    n22 = Index Array(array=w162, index=0 ("line index")) -> (element=w157:string)
    "Command running:" <- w157
    n23 = control-ref of="Interrupt scan"() -> (w181:refnum<vi>)
    n24 = Spreadsheet String To Array(delimiter (Tab)=" ", format string="%s", spreadsheet string=w157, array type (2D Dbl)=string[] []) -> (array=w155:string[])
    n25 = Delete From Array(array=w155, index=0) -> (deleted portion=w104:string, array with subset deleted=w154:string[])  [unwired: 1 in]
    n26 = call "Elapsed Time"("Reset"="Reset", "Auto Reset"="Auto Reset") -> ("Elapsed Time (s)"=w164:dbl)  [unwired: 10 in, 7 out]
    n27 = case shown="2" "Time Units" {
      tunnel: ["-sec" "-min" "-h"] -> w165
      tunnel: [w195 w199 w202] -> w135
      tunnel: w164 -> [w195 w198 w203]
      frame 0, Default {
      }
      frame 1 {
        n28 = Divide(x=w198, y=60.0) -> (x/y=w199:dbl)
      }
      frame 2 {
        n29 = Divide(x=w203, y=3600.0) -> (x/y=w202:dbl)
      }
    }
    n30 = Add(x=w135, y="Time Offset") -> (x+y=w134:dbl)
    n31 = To Long Integer(number=w134) -> (32bit integer=w117:i32)
    "Elapsed Time" <- w117
    n32 = case shown="\"output2\"" w104 {
      tunnel: w154 -> [w235 w268 w300 w428 w451 w588 w678 w826 w899 w926 w996 w1037 w1076 w1111 w1139 _ _ w1285 w1360 _ w1453 w1511 w1567 w1651 w1727 w1761]
      tunnel: w191 -> [w230 w264 w298 w435 w512 w596 w685 w833 w907 w944 w985 w1029 w1069 w1105 w1132 w1165 w1221 w1263 w1342 w1387 w1440 w1498 w1555 w1645 w1723 w1763]
      tunnel: w190 -> [w229 w263 w289 w406 w497 w565 w654 w804 w875 w945 w986 w1030 w1070 w1106 w1133 w1170 w1223 w1291 w1366 w1391 w1459 w1517 w1573 w1657 w1681 w1767]
      tunnel: w189 -> [w228 w262 w288 w405 w496 w564 w651 w803 w872 w946 w987 w1031 w1071 w1107 w1134 w1169 w1194 w1290 w1365 w1390 w1458 w1516 w1572 w1656 w1680 w1766]
      tunnel: w188 -> [w227 w261 w297 w431 w472 w592 w681 w829 w903 w954 w995 w1028 w1068 w1104 w1131 w1168 w1218 w1254 w1334 w1396 w1433 w1491 w1548 w1644 w1722 w1768]
      tunnel: w187 -> [w226 w260 w296 w433 w510 w594 w683 w831 w905 w953 w994 w1036 w1075 w1110 w1138 w1167 w1203 w1289 w1364 w1399 w1457 w1515 w1571 w1655 w1731 w1769]
      tunnel: w186 -> [w225 w259 w295 w432 w509 w593 w682 w830 w904 w952 w993 w1035 w1074 w1109 w1137 w1166 w1204 w1264 w1343 w1398 w1441 w1499 w1556 w1646 w1724 w1771]
      tunnel: [w229 w263 w287 w430 w507 w590 w680 w828 w901 w945 w986 w1030 w1070 w1106 w1133 w1170 w1223 w1255 w1316 w1389 w1434 w1492 w1549 w1597 w1683 w1767] -> w185
      tunnel: [w228 w262 w286 w429 w506 w589 w679 w827 w900 w946 w987 w1031 w1071 w1107 w1134 w1169 w1193 w1265 w1317 w1388 w1442 w1500 w1557 w1596 w1682 w1765] -> w116
      tunnel: [w227 w261 w297 w431 w468 w592 w681 w829 w903 w947 w988 w1028 w1068 w1104 w1131 w1168 w1218 w1254 w1334 w1396 w1433 w1491 w1548 w1644 w1722 w1768] -> w184
      tunnel: [w226 w260 w296 w433 w510 w594 w683 w831 w905 w953 w994 w1036 w1075 w1110 w1138 w1167 w1203 w1289 w1364 w1399 w1457 w1515 w1571 w1655 w1731 w1769] -> w183
      tunnel: [w225 w259 w295 w432 w509 w593 w682 w830 w904 w952 w993 w1035 w1074 w1109 w1137 w1166 w1204 w1264 w1343 w1398 w1441 w1499 w1556 w1646 w1724 w1771] -> w182
      tunnel: [w230 w264 w298 w435 w512 w596 w685 w833 w907 w944 w985 w1029 w1069 w1105 w1132 w1165 w1221 w1263 w1342 w1387 w1440 w1498 w1555 w1645 w1723 w1763] -> w70
      tunnel: w181 -> [_ _ _ w437 w516 w601 w688 w835 w911 _ _ _ _ _ _ _ _ w1260 w1339 _ w1439 w1497 w1554 w1617 w1699 _]
      tunnel: "Gate" -> [_ _ _ w415 w500 w575 w665 w813 w886 _ _ _ _ _ _ _ _ _ _ _ _ _ _ _ _ _]
      tunnel: "Drain 2" -> [_ _ _ w414 w499 w574 w664 w812 w885 _ _ _ _ _ _ _ _ _ _ _ _ _ _ _ _ _]
      tunnel: "Panel Controls" -> [_ _ _ _ _ w573 w663 w702 w884 _ _ _ _ _ _ _ _ _ _ _ _ _ _ _ _ _]
      tunnel: w177 -> [w224 w258 w294 w399 w490 w558 w649 w797 w870 w951 w992 _ w1067 w1103 w1130 w1164 w1205 w1250 w1330 w1392 w1429 w1487 w1544 w1640 w1718 w1772]
      tunnel: w176 -> [w223 w257 w293 w398 w489 w557 w648 w796 w869 w950 w991 w1034 _ w1094 w1136 w1163 w1206 w1251 w1331 w1393 w1430 w1488 w1545 w1641 w1719 w1773]
      tunnel: w175 -> [w222 w256 w292 w397 w488 w556 w647 w795 w868 w949 w990 w1033 w1073 w1108 _ w1162 w1207 w1252 w1332 w1394 w1431 w1489 w1546 w1642 w1720 w1774]
      tunnel: w174 -> [w221 w255 w291 w396 w487 w555 w650 w794 w871 w948 w989 w1032 w1072 _ w1135 w1161 w1208 w1253 w1333 w1395 w1432 w1490 w1547 w1643 w1721 w1775]
      tunnel: [w224 w258 w294 w399 w490 w558 w649 w797 w870 w951 w992 w1027 w1067 w1103 w1130 w1164 w1205 w1250 w1330 w1392 w1429 w1487 w1544 w1640 w1718 w1772] -> w173
      tunnel: [w223 w257 w293 w398 w489 w557 w648 w796 w869 w950 w991 w1034 w1059 w1094 w1136 w1163 w1206 w1251 w1331 w1393 w1430 w1488 w1545 w1641 w1719 w1773] -> w172
      tunnel: [w222 w256 w292 w397 w488 w556 w647 w795 w868 w949 w990 w1033 w1073 w1108 w1129 w1162 w1207 w1252 w1332 w1394 w1431 w1489 w1546 w1642 w1720 w1774] -> w171
      tunnel: [w221 w255 w291 w396 w487 w555 w650 w794 w871 w948 w989 w1032 w1072 w1095 w1135 w1161 w1208 w1253 w1333 w1395 w1432 w1490 w1547 w1643 w1721 w1775] -> w170
      tunnel: w169 -> [_ _ _ w391 w484 _ w643 w789 _ _ _ _ _ _ _ _ _ _ _ _ _ _ _ _ _ _]
      tunnel: w168 -> [_ _ _ w389 w483 _ _ _ _ _ _ _ _ _ _ _ _ _ _ _ _ _ _ _ _ _]
      tunnel: [w220 w251 w284 w321 w460 w545 w640 w720 w857 w943 w983 w1026 w1058 w1093 w1128 w1160 w1189 w1242 w1299 w1386 w1418 w1480 w1538 w1594 w1676 w1764] -> w82
      tunnel: w167 -> [w220 w251 w284 w386 w460 w545 w640 w785 w857 w943 w983 w1026 w1058 w1093 w1128 w1160 w1189 w1242 w1299 w1386 w1418 w1480 w1538 w1594 w1676 w1764]
      tunnel: w134 -> [_ _ _ w383 w457 w543 w638 w782 w854 _ _ _ _ _ _ _ w1187 w1240 w1312 _ w1415 w1477 w1535 w1591 w1672 _]
      tunnel: w165 -> [_ _ _ w380 w456 w541 w637 w779 w853 _ _ _ _ _ _ _ w1185 w1238 w1311 _ w1414 w1476 w1534 w1590 w1673 _]
      tunnel: w117 -> [_ _ _ w375 _ _ _ w774 _ _ _ _ _ _ _ _ _ _ _ _ _ _ _ _ _ _]
      tunnel: [w219 w250 w283 w329 w459 w544 w639 w728 w856 w942 w982 w1025 w1057 w1092 w1127 w1159 w1188 w1241 w1314 w1385 w1417 w1479 w1537 w1593 w1675 w1770] -> w118
      tunnel: w163 -> [w219 w250 w283 w379 w459 w544 w639 w778 w856 w942 w982 w1025 w1057 w1092 w1127 w1159 w1188 w1241 w1314 w1385 w1417 w1479 w1537 w1593 w1675 w1770]
      tunnel: [w218 w249 w282 w320 w455 w540 w636 w719 w852 w941 w981 w1024 w1056 w1091 w1126 w1158 w1184 w1237 w1298 w1384 w1413 w1475 w1533 w1589 w1671 w1759] -> w81
      tunnel: w139 -> [w218 w249 w282 w373 w455 w540 w636 w772 w852 w941 w981 w1024 w1056 w1091 w1126 w1158 w1184 w1237 w1298 w1384 w1413 w1475 w1533 w1589 w1671 w1759]
      tunnel: [w217 w248 w281 w366 w454 w539 w626 w765 w851 w940 w980 w1023 w1055 w1090 w1125 w1157 w1183 w1236 w1310 w1383 w1412 w1474 w1532 w1588 w1670 w1758] -> w112
      tunnel: w125 -> [w217 w248 w281 w366 w454 w539 w626 w765 w851 w940 w980 w1023 w1055 w1090 w1125 w1157 w1183 w1236 w1310 w1383 w1412 w1474 w1532 w1588 w1670 w1757]
      tunnel: [w216 w247 w280 w365 w453 w538 w625 w764 w850 w939 w979 w1022 w1054 w1089 w1124 w1156 w1182 w1235 w1309 w1382 w1411 w1473 w1531 w1587 w1669 w1743] -> w120
      tunnel: w119 -> [w216 w247 w280 w365 w453 w538 w625 w764 w850 w939 w979 w1022 w1054 w1089 w1124 w1156 w1182 w1235 w1309 w1382 w1411 w1473 w1531 w1587 w1669 w1743]
      tunnel: w117 -> [_ _ _ _ _ _ _ _ _ _ _ _ _ _ _ _ _ _ _ _ _ _ _ _ _ _]
      tunnel: [w215 w246 w279 w364 w452 w537 w624 w763 w849 w938 w978 w1021 w1053 w1088 w1123 w1155 w1181 w1234 w1308 w1381 w1410 w1472 w1530 w1586 w1668 w1742] -> w113
      tunnel: w115 -> [w215 w246 w279 w364 w452 w537 w624 w763 w849 w938 w978 w1021 w1053 w1088 w1123 w1155 w1181 w1234 w1308 w1381 w1410 w1472 w1530 w1586 w1668 w1742]
      tunnel: [w213 w244 w277 w314 w449 w535 w622 w713 w847 w936 w977 w1020 w1051 w1086 w1121 w1153 w1179 w1233 w1307 w1380 w1409 w1471 w1528 w1585 w1667 w1741] -> w75
      tunnel: w103 -> [w213 w244 w277 w360 w449 w535 w622 w759 w847 w936 w977 w1020 w1051 w1086 w1121 w1153 w1179 w1233 w1307 w1380 w1409 w1471 w1528 w1585 w1667 w1741]
      tunnel: [w214 w245 w278 w315 w450 w536 w623 w714 w848 w937 w976 w1019 w1052 w1087 w1122 w1154 w1180 w1232 w1306 w1379 w1408 w1470 w1529 w1584 w1666 w1740] -> w76
      tunnel: w102 -> [w214 w245 w278 w359 w450 w536 w623 w758 w848 w937 w976 w1019 w1052 w1087 w1122 w1154 w1180 w1232 w1306 w1379 w1408 w1470 w1529 w1584 w1666 w1740]
      tunnel: [w206 w237 w270 w319 w446 w533 w620 w718 w845 w929 w974 w1017 w1049 w1084 w1119 w1151 w1172 w1225 w1297 w1378 w1401 w1463 w1521 w1577 w1661 w1733] -> w80
      tunnel: w91 -> [w206 w237 w270 w349 w446 w533 w620 w748 w845 w929 w974 w1017 w1049 w1084 w1119 w1151 w1172 w1225 w1297 w1378 w1401 w1463 w1521 w1577 w1661 w1733]
      tunnel: [w205 w236 w269 w318 w447 w534 w621 w717 w846 w928 w975 w1018 w1050 w1085 w1120 w1152 w1171 w1224 w1296 w1377 w1400 w1462 w1520 w1576 w1660 w1732] -> w79
      tunnel: w90 -> [w205 w236 w269 w348 w447 w534 w621 w747 w846 w928 w975 w1018 w1050 w1085 w1120 w1152 w1171 w1224 w1296 w1377 w1400 w1462 w1520 w1576 w1660 w1732]
      tunnel: [w208 w239 w272 w324 w445 w531 w618 w723 w843 w934 w972 w1015 w1047 w1082 w1117 w1149 w1174 w1227 w1301 w1372 w1403 w1465 w1523 w1579 w1659 w1737] -> w73
      tunnel: w89 -> [w208 w239 w272 w345 w445 w531 w618 w744 w843 w934 w972 w1015 w1047 w1082 w1117 w1149 w1174 w1227 w1301 w1372 w1403 w1465 w1523 w1579 w1659 w1737]
      tunnel: [w207 w238 w271 w322 w448 w532 w619 w721 w844 w935 w973 w1016 w1048 w1083 w1118 w1150 w1173 w1226 w1300 w1371 w1402 w1464 w1522 w1578 w1658 w1736] -> w83
      tunnel: w88 -> [w207 w238 w271 w344 w448 w532 w619 w743 w844 w935 w973 w1016 w1048 w1083 w1118 w1150 w1173 w1226 w1300 w1371 w1402 w1464 w1522 w1578 w1658 w1736]
      tunnel: [w210 w241 w274 w313 w444 w529 w616 w712 w841 w932 w970 w1013 w1045 w1080 w1115 w1147 w1176 w1229 w1303 w1374 w1405 w1467 w1525 w1581 w1663 w1739] -> w74
      tunnel: w87 -> [w210 w241 w274 w341 w444 w529 w616 w740 w841 w932 w970 w1013 w1045 w1080 w1115 w1147 w1176 w1229 w1303 w1374 w1405 w1467 w1525 w1581 w1663 w1739]
      tunnel: [w209 w240 w273 w312 w443 w530 w617 w711 w842 w933 w971 w1014 w1046 w1081 w1116 w1148 w1175 w1228 w1302 w1373 w1404 w1466 w1524 w1580 w1662 w1738] -> w72
      tunnel: w86 -> [w209 w240 w273 w340 w443 w530 w617 w739 w842 w933 w971 w1014 w1046 w1081 w1116 w1148 w1175 w1228 w1302 w1373 w1404 w1466 w1524 w1580 w1662 w1738]
      tunnel: [w212 w243 w276 w317 w442 w527 w614 w716 w839 w930 w968 w1011 w1043 w1078 w1113 w1145 w1178 w1231 w1305 w1376 w1407 w1469 w1527 w1583 w1665 w1735] -> w78
      tunnel: w85 -> [w212 w243 w276 w337 w442 w527 w614 w736 w839 w930 w968 w1011 w1043 w1078 w1113 w1145 w1178 w1231 w1305 w1376 w1407 w1469 w1527 w1583 w1665 w1735]
      tunnel: [w211 w242 w275 w316 w441 w528 w615 w715 w840 w931 w969 w1012 w1044 w1079 w1114 w1146 w1177 w1230 w1304 w1375 w1406 w1468 w1526 w1582 w1664 w1734] -> w77
      tunnel: w84 -> [w211 w242 w275 w336 w441 w528 w615 w735 w840 w931 w969 w1012 w1044 w1079 w1114 w1146 w1177 w1230 w1304 w1375 w1406 w1468 w1526 w1582 w1664 w1734]
      frame "wait" {
        n33 = Index Array(array=w235, index=0 ("Index")) -> (element=w233:string)
        n34 = Decimal String To Number(string=w233, default (0L)=u32 0) -> (number=w232:u32)  [unwired: 1 in, 1 out]
        n35 = Wait (ms)(milliseconds to wait=w232) -> ()  [unwired: 1 out]
      }
      frame "wait-min" {
        n36 = Index Array(array=w268, index=0 ("Index")) -> (element=w266:string)
        n37 = Decimal String To Number(string=w266, default (0L)=u32 0) -> (number=w254:u32)  [unwired: 1 in, 1 out]
        n38 = Multiply(x=w254, y=u32 60000) -> (x*y=w253:u32)
        n39 = Wait (ms)(milliseconds to wait=w253) -> ()  [unwired: 1 out]
      }
      frame "standby" {
        n40 = Index Array(array=w300, index=0 ("Index")) -> (element=w290:string)
        n41 = case shown="\"off\", Default" w290 {
          tunnel: [":PAGE:SCON:STAN 0" ":PAGE:SCON:STAN 1"] -> w285
          frame "off", Default {
          }
          frame "on" {
          }
        }
        n42 = VISA Write(VISA resource name=w289, write buffer=w285, error in (no error)=w288) -> (VISA resource name out=w287:refnum<visa-resource-name>, error out=w286:errorcluster)  [unwired: 1 out]
      }
      frame "transfer" {
        # "Adjusts graph colors."
        # "Adjusts graph colors."
        # "Is off"
        # "Is on"
        # "Ion will be the middle element of the array. The calculation of the index is done only once, since Is, Id, and Ig have the same dimensions."
        # "Ig off"
        # "Ig on"
        # "Is min"
        # "Is max"
        # "Ig min"
        # "Ig max"
        # "abs(Ig)"
        # "abs(Is)"
        # "Id min"
        # "Id max"
        # "Y1: Is\nY2: Id\nY3: Ig"
        # "abs(Id)"
        # "Adjusts graph colors."
        # "Adjusts graph colors."
        # "Id off"
        # "Id on"
        # "Adjusts graph colors."
        # "Time array"
        n43 = Delete From Array(array=w428, index=0 ("Index")) -> (deleted portion=w426:string, array with subset deleted=w425:string[])  [unwired: 1 in]
        n44 = Bundle By Name(cluster=w389, "Emergency Stop"=w437) -> (w390:T3)
        n45 = Number To Decimal String(number=w383) -> (decimal integer string=w382:string)  [unwired: 1 in]
        n46 = case shown="\"d\", Default" w426 {
          tunnel: [w439 w440] -> w424
          frame "s" {
            w439 = u16 0 items=["Single", "Double"] ("sweep mode")
          }
          frame "d", Default {
            w440 = u16 1 items=["Single", "Double"] ("sweep mode")
          }
        }
        n47 = Fract/Exp String To Number(string=w425) -> (number=w410:dbl[])  [unwired: 3 in, 1 out]
        n48 = Concatenate Strings(w435, "-transfer-" ("Prefix"), w382, w380, ".txt" ("Suffix (transfer)")) -> (w436:string)
        n49 = VISA Write(VISA resource name=w406, write buffer=":PAGE:CHAN:MODE SWE;" ("write buffer (\"\")"), error in (no error)=w405) -> (VISA resource name out=w403:refnum<visa-resource-name>, error out=w404:errorcluster)  [unwired: 1 out]
        n50 = String To Path(string=w436) -> (path=w434:path)
        n51 = Index Array(array=w410, index #1=0 ("Index")) -> (element #1=w423:dbl, element #2=w422:dbl, element #3=w421:dbl)  [unwired: 2 in]
        n52 = Delete From Array(array=w410, length=3 ("Length"), index=0 ("Index")) -> (array with subset deleted=w408:dbl[])  [unwired: 1 out]
        n53 = Build Array (concatenate)(w379, w375) -> (w329:i32[])
        n54 = Bundle By Name(cluster=w415, "Gate Start"=w423, "Gate Stop"=w422, "Gate Step (linear only)"=w421, "Gate Compliance"=w432, "Range mode"=w399, "Range"=w398) -> (w400:T6)
        n55 = control-ref of="Imax vs time"() -> (w358:refnum<vi>)
        n56 = control-ref of="Imin vs time"() -> (w357:refnum<vi>)
        n57 = control-ref of="Ion vs time"() -> (w326:refnum<vi>)
        n58 = control-ref of="Ioff vs time"() -> (w325:refnum<vi>)
        n59 = control-ref of="I vs Vg"() -> (w384:refnum<vi>)
        n60 = Index Array(array=w408, index #1=0 ("Index")) -> (element #1=w418:dbl, element #2=w417:dbl, element #3=w416:dbl)  [unwired: 2 in]
        n61 = call <vilib>:"compatOverwrite.vi"("overwrite (F)"=TRUE) -> ("overwrite?"=w388:T8)
        n62 = Bundle By Name(cluster=w414, "Drain Start"=w418, "Drain Stop"=w417, "Drain Step"=w416, "Drain Compliance"=w433, "Range mode"=w397, "Range"=w396) -> (w401:T7)
        n63 = call "4155C Transfer.vi"("VISA resource name in"=w403, "Gate"=w400, "Drain"=w401, "Timings"=w431, "error in (no error)"=w404, "SMU4"=w391, "sweep mode"=w424, "Panel Controls"=w390) -> ("VG"=w387:dbl[], "Outparams"=w395:T9, "VISA Resource Name out"=w430:refnum<visa-resource-name>, "IS"=w354:dbl[], "ID"=w356:dbl[], "IG"=w353:dbl[], "error out"=w376:errorcluster, "SMU4"=w392:dbl[])  [unwired: 12 in]
        n64 = Unbundle By Name(w395) -> ("V2 Step"=w394:dbl, "V2 Start"=w393:dbl, "Number of points"=w323:i32)
        n65 = Absolute Value(x=w354) -> (abs(x)=w339:dbl[])
        n66 = Absolute Value(x=w356) -> (abs(x)=w355:dbl[])
        n67 = Absolute Value(x=w353) -> (abs(x)=w342:dbl[])
        n68 = Array Size(array=w355) -> (size(s)=w363:i32)
        n69 = Divide(x=w363, y=2) -> (x/y=w306:dbl)
        n70 = Subtract(x=w306, y=1) -> (x-y=w305:dbl)
        n71 = Array Max & Min(array=w339) -> (max value=w346:dbl, min value=w347:dbl)  [unwired: 2 out]
        n72 = Array Max & Min(array=w355) -> (max value=w385:dbl, min value=w352:dbl)  [unwired: 2 out]
        n73 = Array Max & Min(array=w342) -> (max value=w351:dbl, min value=w350:dbl)  [unwired: 2 out]
        n74 = call "4155C Split array.vi"("Number of VAR2 steps"=w323, "Y2 data in"=w356, "X data in"=w387, "Y1 data in"=w354, "Y3 data in"=w353, "error in (no error)"=w376) -> ("Array of clusters"=w378:cluster{"Y data in":dbl[], "X data in":dbl[]}[], "error out"=w311:errorcluster)  [unwired: 1 in]
        n75 = Index Array(array=w339, index=w305) -> (element=w330:dbl)
        n76 = Index Array(array=w339, index=0) -> (element=w331:dbl)
        n77 = Index Array(array=w355, index=w305) -> (element=w332:dbl)
        n78 = Index Array(array=w355, index=0) -> (element=w333:dbl)
        n79 = Index Array(array=w342, index=w305) -> (element=w335:dbl)
        n80 = Index Array(array=w342, index=0) -> (element=w334:dbl)
        n81 = local write "Ig max"(w351) -> ()
        n82 = local write "Ig min"(w350) -> ()
        n83 = local write "Is max"(w346) -> ()
        n84 = local write "Is min"(w347) -> ()
        n85 = local write "Id max"(w385) -> ()
        n86 = local write "Id min"(w352) -> ()
        n87 = local write "I vs Vg"(w378) -> ()
        n88 = Build Array (concatenate)(w345, w346) -> (w324:dbl[])
        n89 = Build Array (concatenate)(w344, w347) -> (w322:dbl[])
        n90 = local write "Is off"(w331) -> ()
        n91 = local write "Is on"(w330) -> ()
        n92 = Build Array (concatenate)(w386, w385) -> (w321:dbl[])
        n93 = Build Array (concatenate)(w373, w352) -> (w320:dbl[])
        n94 = Build Array (concatenate)(w349, w351) -> (w319:dbl[])
        n95 = Build Array (concatenate)(w348, w350) -> (w318:dbl[])
        n96 = Build Array (concatenate)(w337, w330) -> (w317:dbl[])
        n97 = Build Array (concatenate)(w336, w331) -> (w316:dbl[])
        n98 = Build Array (concatenate)(w359, w332) -> (w315:dbl[])
        n99 = Build Array (concatenate)(w360, w333) -> (w314:dbl[])
        n100 = Build Array (concatenate)(w341, w335) -> (w313:dbl[])
        n101 = Build Array (concatenate)(w340, w334) -> (w312:dbl[])
        n102 = local write "Ig off"(w334) -> ()
        n103 = local write "Ig on"(w335) -> ()
        n104 = local write "Id off"(w333) -> ()
        n105 = local write "Id on"(w332) -> ()
        n106 = call "4155C Split array.vi"("Number of VAR2 steps"=w323, "Y2 data in"=w315, "X data in"=w329, "Y1 data in"=w317, "Y3 data in"=w313, "error in (no error)"=w311) -> ("Array of clusters"=w327:cluster{"Y data in":dbl[], "X data in":dbl[]}[], "error out"=w310:errorcluster)  [unwired: 1 in]
        n107 = call "4155C Split array.vi"("Number of VAR2 steps"=w323, "Y2 data in"=w314, "X data in"=w329, "Y1 data in"=w316, "Y3 data in"=w312, "error in (no error)"=w310) -> ("Array of clusters"=w328:cluster{"Y data in":dbl[], "X data in":dbl[]}[], "error out"=w309:errorcluster)  [unwired: 1 in]
        n108 = call "4155C Split array.vi"("Number of VAR2 steps"=w323, "Y2 data in"=w321, "X data in"=w329, "Y1 data in"=w324, "Y3 data in"=w319, "error in (no error)"=w309) -> ("Array of clusters"=w377:cluster{"Y data in":dbl[], "X data in":dbl[]}[], "error out"=w308:errorcluster)  [unwired: 1 in]
        n109 = call "4155C Split array.vi"("Number of VAR2 steps"=w323, "Y2 data in"=w320, "X data in"=w329, "Y1 data in"=w322, "Y3 data in"=w318, "error in (no error)"=w308) -> ("Array of clusters"=w374:cluster{"Y data in":dbl[], "X data in":dbl[]}[], "error out"=w307:errorcluster)  [unwired: 1 in]
        n110 = Open/Create/Replace File(file path (use dialog)=w434, error in=w307, operation (0:open)=w388) -> (refnum out=w371:refnum<file>, error out=w369:errorcluster)  [unwired: 3 in, 1 out]
        n111 = call "4155C Make Big 2d array.vi"("1D Var1"=w387, "1d IS"=w354, "1d ID"=w356, "1d IG"=w353, "1d SMU4"=w392, "SMU4"=w391, "VAR2 START"=w393, "Number of VAR2 steps"=w323, "VAR2 STEP"=w394, "VAR1 Name"="Vg", "Decimal places in header"=i8 1, "VAR2 Name"="Vd") -> ("Header array"=w372:string[], "Data array"=w370:dbl[][])  [unwired: 14 in]
        n112 = local write "Imax vs time"(w377) -> ()
        n113 = local write "Imin vs time"(w374) -> ()
        n114 = local write "Ion vs time"(w327) -> ()
        n115 = local write "Ioff vs time"(w328) -> ()
        n116 = call "4155C Config Chart Colours.vi"("Numeric"=w323, "XY Graph 2"=w358) -> ()  [unwired: 6 in]
        n117 = call "4155C Config Chart Colours.vi"("Numeric"=w323, "XY Graph 2"=w357) -> ()  [unwired: 6 in]
        n118 = call "4155C Config Chart Colours.vi"("Numeric"=w323, "XY Graph 2"=w326) -> ()  [unwired: 6 in]
        n119 = call "4155C Config Chart Colours.vi"("Numeric"=w323, "XY Graph 2"=w325) -> ()  [unwired: 6 in]
        n120 = call "4155C Config Chart Colours.vi"("Numeric"=w323, "XY Graph 2"=w384) -> ()  [unwired: 6 in]
        n121 = call "4155C Write array to file.vi"("Byte Stream File Refnum"=w371, "Header"=w372, "Data Array"=w370, "error in (no error)"=w369) -> ("dup refnum"=w368:refnum<file>, "error out"=w367:errorcluster)  [unwired: 1 in]
        n122 = Close File(refnum=w368, error in=w367) -> (error out=w429:errorcluster)  [unwired: 1 out]
      }
      frame "pulsedstressV" {
        w466 = 0
        n123 = Number To Decimal String(number=w457) -> (decimal integer string=w513:string)  [unwired: 1 in]
        n124 = Delete From Array(array=w451, index=0 ("Index")) -> (deleted portion=w504:string, array with subset deleted=w503:string[])  [unwired: 1 in]
        n125 = Bundle By Name(cluster=w483, "Emergency Stop"=w516) -> (w485:T3)
        n126 = VISA Write(VISA resource name=w497, write buffer=":PAGE:CHAN:MODE SWE;" ("write buffer (\"\")"), error in (no error)=w496) -> (VISA resource name out=w494:refnum<visa-resource-name>, error out=w495:errorcluster)  [unwired: 1 out]
        n127 = Concatenate Strings(w512, "-pulsedstressV-" ("Substring"), w513, w456, ".txt" ("Substring")) -> (w515:string)
        n128 = case shown="\"d\", Default" w504 {
          tunnel: [w525 w526] -> w502
          frame "s" {
            w525 = u16 0 items=["Single", "Double"] ("sweep mode")
          }
          frame "d", Default {
            w526 = u16 1 items=["Single", "Double"] ("sweep mode")
          }
        }
        n129 = Fract/Exp String To Number(string=w503) -> (number=w498:dbl[])  [unwired: 3 in, 1 out]
        n130 = String To Path(string=w515) -> (path=w511:path)
        n131 = Index Array(array=w498, index #1=0 ("Index")) -> (element #1=w475:dbl, element #2=w474:dbl, element #3=w471:dbl, element #4=w470:dbl, element #5=w469:dbl, element #6=w473:dbl)  [unwired: 5 in]
        n132 = Bundle By Name(cluster=w472, "Pulse period"=w470, "Base voltage"=w471, "Pulse width"=w469) -> (w468:T5)
        n133 = Unbundle By Name(w468) -> ("Pulse period"=w476:dbl)
        n134 = Bundle By Name(cluster=w500, "Gate Start"=w474, "Gate Stop"=w475, "Gate Step (linear only)"=0, "Gate Compliance"=w509, "Range mode"=w490, "Range"=w489) -> (w491:T6)
        n135 = call <vilib>:"compatOverwrite.vi"("overwrite (F)"=TRUE) -> ("overwrite?"=w461:T8)
        n136 = Bundle By Name(cluster=w499, "Drain Start"=w473, "Drain Stop"=w466, "Drain Step"=w466, "Drain Compliance"=w510, "Range mode"=w488, "Range"=w487) -> (w492:T7)
        n137 = call "4155C PulsedStressV.vi"("VISA resource name in"=w494, "sweep mode"=w502, "Panel Controls"=w485, "Gate"=w491, "Drain"=w492, "Timings"=w468, "error in (no error)"=w495, "SMU4"=w484) -> ("VISA Resource Name out"=w507:refnum<visa-resource-name>, "ID"=w464:dbl[], "IG"=w462:dbl[], "Outparams"=w486:T9, "error out"=w508:errorcluster)  [unwired: 3 in]
        n138 = Unbundle By Name(w486) -> ("Number of points"=w463:i32)  [unwired: 2 out]
        n139 = for {
          N: w463 -> [_]
          tunnel: [w522] -> w465 mode=indexing
          tunnel: w476 -> [w524]
          i -> [w523]
          n140 = Multiply(x=w524, y=w523) -> (x*y=w522:dbl)
        }
        n141 = Insert Into Array(array=dbl[][] [] ("Input Array"), new element=w465) -> (w477:dbl[][])  [unwired: 2 in]
        n142 = Insert Into Array(array=w477, new element=w464) -> (w482:dbl[][])  [unwired: 2 in]
        n143 = Insert Into Array(array=w482, new element=w462) -> (w481:dbl[][])  [unwired: 2 in]
        n144 = Transpose 2D Array(2D array=w481) -> (transposed array=w480:dbl[][])
        n145 = Open/Create/Replace File(file path (use dialog)=w511, error in=w508, operation (0:open)=w461) -> (refnum out=w519:refnum<file>, error out=w520:errorcluster)  [unwired: 3 in, 1 out]
        n146 = call "4155C Write array to file.vi"("Byte Stream File Refnum"=w519, "Header"=string[] ["Time /s", "Id /A", "Ig /A"], "Data Array"=w480, "error in (no error)"=w520) -> ("dup refnum"=w517:refnum<file>, "error out"=w518:errorcluster)  [unwired: 1 in]
        n147 = Close File(refnum=w517, error in=w518) -> (error out=w506:errorcluster)  [unwired: 1 out]
      }
      frame "transfer-fpp" {
        n148 = Number To Decimal String(number=w543) -> (decimal integer string=w597:string)  [unwired: 1 in]
        n149 = Bundle By Name(cluster=w573, "Emergency Stop"=w601) -> (w609:T2)
        n150 = Delete From Array(array=w588, index=0 ("Index")) -> (deleted portion=w586:string, array with subset deleted=w585:string[])  [unwired: 1 in]
        n151 = Concatenate Strings(w596, "-transferfpp-" ("Substring"), w597, w541, ".txt" ("Substring")) -> (w599:string)
        n152 = VISA Write(VISA resource name=w565, write buffer=":PAGE:CHAN:MODE SWE;" ("write buffer (\"\")"), error in (no error)=w564) -> (VISA resource name out=w562:refnum<visa-resource-name>, error out=w563:errorcluster)  [unwired: 1 out]
        n153 = case shown="\"d\", Default" w586 {
          tunnel: [w610 w611] -> w584
          frame "s" {
            w610 = u16 0 items=["Single", "Double"] ("sweep mode")
          }
          frame "d", Default {
            w611 = u16 1 items=["Single", "Double"] ("sweep mode")
          }
        }
        n154 = Fract/Exp String To Number(string=w585) -> (number=w569:dbl[])  [unwired: 3 in, 1 out]
        n155 = String To Path(string=w599) -> (path=w595:path)
        n156 = Index Array(array=w569, index #1=0 ("Index")) -> (element #1=w583:dbl, element #2=w582:dbl, element #3=w581:dbl)  [unwired: 2 in]
        n157 = Delete From Array(array=w569, length=3 ("Length"), index=0 ("Index")) -> (array with subset deleted=w567:dbl[])  [unwired: 1 out]
        n158 = Bundle By Name(cluster=w575, "Gate Start"=w583, "Gate Stop"=w582, "Gate Step (linear only)"=w581, "Gate Compliance"=w593, "Range mode"=w558, "Range"=w557) -> (w559:T6)
        n159 = Index Array(array=w567, index #1=0 ("Index")) -> (element #1=w578:dbl, element #2=w577:dbl, element #3=w576:dbl)  [unwired: 2 in]
        n160 = call <vilib>:"compatOverwrite.vi"("overwrite (F)"=TRUE) -> ("overwrite?"=w546:T8)
        n161 = Bundle By Name(cluster=w574, "Drain Start"=w578, "Drain Stop"=w577, "Drain Step"=w576, "Drain Compliance"=w594, "Range mode"=w556, "Range"=w555) -> (w560:T7)
        n162 = call "4155C Transfer-FPP.vi"("VISA resource name in"=w562, "Gate"=w559, "Drain"=w560, "Timings"=w592, "error in (no error)"=w563, "sweep mode"=w584, "Panel Controls"=w609) -> ("VG"=w600:dbl[], "Outparams"=w554:T9, "VISA Resource Name out"=w590:refnum<visa-resource-name>, "Vprobe2"=w550:dbl[], "ID"=w549:dbl[], "IG"=w548:dbl[], "Vprobe1"=w547:dbl[], "error out"=w591:errorcluster)  [unwired: 13 in]
        n163 = Unbundle By Name(w554) -> ("V2 Step"=w553:dbl, "V2 Start"=w552:dbl, "Number of points"=w551:i32)
        n164 = Open/Create/Replace File(file path (use dialog)=w595, error in=w591, operation (0:open)=w546) -> (refnum out=w606:refnum<file>, error out=w607:errorcluster)  [unwired: 3 in, 1 out]
        n165 = call "4155C Make Big 2d array FPP.vi"("1D Var1"=w600, "1d ID"=w549, "1d Vp2"=w550, "1d IG"=w548, "1d Vp1"=w547, "VAR2 START"=w552, "Number of VAR2 steps"=w551, "VAR2 STEP"=w553, "VAR1 Name"="Vg", "Decimal places in header"=i8 1, "VAR2 Name"="Vd") -> ("Header array"=w602:string[], "Data array"=w603:dbl[][])  [unwired: 15 in]
        n166 = call "4155C Write array to file.vi"("Byte Stream File Refnum"=w606, "Header"=w602, "Data Array"=w603, "error in (no error)"=w607) -> ("dup refnum"=w604:refnum<file>, "error out"=w605:errorcluster)  [unwired: 1 in]
        n167 = Close File(refnum=w604, error in=w605) -> (error out=w589:errorcluster)  [unwired: 1 out]
      }
      frame "output" {
        n168 = Number To Decimal String(number=w638) -> (decimal integer string=w686:string)  [unwired: 1 in]
        n169 = Bundle By Name(cluster=w663, "Emergency Stop"=w688) -> (w698:T2)
        n170 = Delete From Array(array=w678, index=0 ("Index")) -> (deleted portion=w676:string, array with subset deleted=w675:string[])  [unwired: 1 in]
        n171 = Concatenate Strings(w685, "-output-" ("Substring"), w686, w637, ".txt" ("Suffix (output)")) -> (w687:string)
        n172 = VISA Write(VISA resource name=w654, write buffer=":PAGE:CHAN:MODE SWE;" ("write buffer (\"\")"), error in (no error)=w651) -> (VISA resource name out=w653:refnum<visa-resource-name>, error out=w652:errorcluster)  [unwired: 1 out]
        n173 = case shown="\"d\", Default" w676 {
          tunnel: [w699 w700] -> w674
          frame "s" {
            w699 = u16 0 items=["Single", "Double"] ("sweep mode")
          }
          frame "d", Default {
            w700 = u16 1 items=["Single", "Double"] ("sweep mode")
          }
        }
        n174 = Fract/Exp String To Number(string=w675) -> (number=w657:dbl[])  [unwired: 3 in, 1 out]
        n175 = String To Path(string=w687) -> (path=w684:path)
        n176 = Index Array(array=w657, index #1=0 ("Index")) -> (element #1=w673:dbl, element #2=w672:dbl, element #3=w671:dbl)  [unwired: 2 in]
        n177 = Delete From Array(array=w657, length=3 ("Length"), index=0 ("Index")) -> (array with subset deleted=w656:dbl[])  [unwired: 1 out]
        n178 = control-ref of="I vs Vd"() -> (w628:refnum<vi>)
        n179 = Bundle By Name(cluster=w665, "Gate Start"=w673, "Gate Stop"=w672, "Gate Step (linear only)"=w671, "Gate Compliance"=w682, "Range mode"=w649, "Range"=w648) -> (w697:T6)
        n180 = Index Array(array=w656, index #1=0 ("Index")) -> (element #1=w668:dbl, element #2=w667:dbl, element #3=w666:dbl)  [unwired: 2 in]
        n181 = call <vilib>:"compatOverwrite.vi"("overwrite (F)"=TRUE) -> ("overwrite?"=w641:T8)
        n182 = Bundle By Name(cluster=w664, "Drain Start"=w668, "Drain Stop"=w667, "Drain Step"=w666, "Drain Compliance"=w683, "Range mode"=w647, "Range"=w650) -> (w696:T7)
        n183 = call "4155C Output.vi"("VISA resource name in"=w653, "Gate"=w697, "Drain"=w696, "Timings"=w681, "error in (no error)"=w652, "SMU4"=w643, "sweep mode"=w674, "Panel controls"=w698) -> ("VD"=w635:dbl[], "Outparams"=w645:T9, "VISA Resource Name out"=w680:refnum<visa-resource-name>, "IS"=w634:dbl[], "ID"=w633:dbl[], "IG"=w632:dbl[], "error out"=w630:errorcluster, "SMU4"=w642:dbl[])  [unwired: 12 in]
        n184 = Unbundle By Name(w645) -> ("V2 Step"=w646:dbl, "V2 Start"=w644:dbl, "Number of points"=w627:i32)
        n185 = call "4155C Split array.vi"("Number of VAR2 steps"=w627, "Y2 data in"=w633, "X data in"=w635, "Y1 data in"=w634, "Y3 data in"=w632, "error in (no error)"=w630) -> ("Array of clusters"=w631:cluster{"Y data in":dbl[], "X data in":dbl[]}[], "error out"=w629:errorcluster)  [unwired: 1 in]
        n186 = local write "I vs Vd"(w631) -> ()
        n187 = call "4155C Config Chart Colours.vi"("Numeric"=w627, "XY Graph 2"=w628) -> ()  [unwired: 6 in]
        n188 = Open/Create/Replace File(file path (use dialog)=w684, error in=w629, operation (0:open)=w641) -> (refnum out=w693:refnum<file>, error out=w694:errorcluster)  [unwired: 3 in, 1 out]
        n189 = call "4155C Make Big 2d array.vi"("1D Var1"=w635, "1d IS"=w634, "1d ID"=w633, "1d IG"=w632, "1d SMU4"=w642, "SMU4"=w643, "VAR2 START"=w644, "Number of VAR2 steps"=w627, "VAR2 STEP"=w646, "VAR1 Name"="Vd", "Decimal places in header"=i8 1, "VAR2 Name"="Vg") -> ("Header array"=w689:string[], "Data array"=w690:dbl[][])  [unwired: 14 in]
        n190 = call "4155C Write array to file.vi"("Byte Stream File Refnum"=w693, "Header"=w689, "Data Array"=w690, "error in (no error)"=w694) -> ("dup refnum"=w691:refnum<file>, "error out"=w692:errorcluster)  [unwired: 1 in]
        n191 = Close File(refnum=w691, error in=w692) -> (error out=w679:errorcluster)  [unwired: 1 out]
      }
      frame "output2" {
        # "Adjusts graph colors."
        # "Adjusts graph colors."
        # "Is off"
        # "Is on"
        # "Ion will be the middle element of the array. The calculation of the index is done only once, since Is, Id, and Ig have the same dimensions."
        # "Ig off"
        # "Ig on"
        # "Is min"
        # "Is max"
        # "Ig min"
        # "Ig max"
        # "abs(Ig)"
        # "abs(Is)"
        # "Id min"
        # "Id max"
        # "Y1: Is\nY2: Id\nY3: Ig"
        # "abs(Id)"
        # "Adjusts graph colors."
        # "Adjusts graph colors."
        # "Id off"
        # "Id on"
        # "Adjusts graph colors."
        # "Time array"
        n192 = Delete From Array(array=w826, index=0 ("Index")) -> (deleted portion=w824:string, array with subset deleted=w823:string[])  [unwired: 1 in]
        n193 = Bundle By Name(cluster=w702, "Emergency Stop"=w835) -> (w788:T2)
        n194 = Number To Decimal String(number=w782) -> (decimal integer string=w781:string)  [unwired: 1 in]
        n195 = case shown="\"d\", Default" w824 {
          tunnel: [w837 w838] -> w822
          frame "s" {
            w837 = u16 0 items=["Single", "Double"] ("sweep mode")
          }
          frame "d", Default {
            w838 = u16 1 items=["Single", "Double"] ("sweep mode")
          }
        }
        n196 = Fract/Exp String To Number(string=w823) -> (number=w808:dbl[])  [unwired: 3 in, 1 out]
        n197 = Concatenate Strings(w833, "-output-" ("Substring"), w781, w779, ".txt" ("Suffix (transfer)")) -> (w834:string)
        n198 = VISA Write(VISA resource name=w804, write buffer=":PAGE:CHAN:MODE SWE;" ("write buffer (\"\")"), error in (no error)=w803) -> (VISA resource name out=w801:refnum<visa-resource-name>, error out=w802:errorcluster)  [unwired: 1 out]
        n199 = String To Path(string=w834) -> (path=w832:path)
        n200 = Index Array(array=w808, index #1=0 ("Index")) -> (element #1=w821:dbl, element #2=w820:dbl, element #3=w819:dbl)  [unwired: 2 in]
        n201 = Delete From Array(array=w808, length=3 ("Length"), index=0 ("Index")) -> (array with subset deleted=w806:dbl[])  [unwired: 1 out]
        n202 = Build Array (concatenate)(w778, w774) -> (w728:i32[])
        n203 = Bundle By Name(cluster=w813, "Gate Start"=w821, "Gate Stop"=w820, "Gate Step (linear only)"=w819, "Gate Compliance"=w830, "Range mode"=w797, "Range"=w796) -> (w798:T6)
        n204 = control-ref of="Imax vs time"() -> (w757:refnum<vi>)
        n205 = control-ref of="Imin vs time"() -> (w756:refnum<vi>)
        n206 = control-ref of="Ion vs time"() -> (w725:refnum<vi>)
        n207 = control-ref of="Ioff vs time"() -> (w724:refnum<vi>)
        n208 = control-ref of="I vs Vg"() -> (w783:refnum<vi>)
        n209 = Index Array(array=w806, index #1=0 ("Index")) -> (element #1=w816:dbl, element #2=w815:dbl, element #3=w814:dbl)  [unwired: 2 in]
        n210 = call <vilib>:"compatOverwrite.vi"("overwrite (F)"=TRUE) -> ("overwrite?"=w787:T8)
        n211 = Bundle By Name(cluster=w812, "Drain Start"=w816, "Drain Stop"=w815, "Drain Step"=w814, "Drain Compliance"=w831, "Range mode"=w795, "Range"=w794) -> (w799:T7)
        n212 = call "4155C Output.vi"("VISA resource name in"=w801, "Gate"=w798, "Drain"=w799, "Timings"=w829, "error in (no error)"=w802, "SMU4"=w789, "sweep mode"=w822, "Panel controls"=w788) -> ("VD"=w786:dbl[], "Outparams"=w793:T9, "VISA Resource Name out"=w828:refnum<visa-resource-name>, "IS"=w753:dbl[], "ID"=w755:dbl[], "IG"=w752:dbl[], "error out"=w775:errorcluster, "SMU4"=w790:dbl[])  [unwired: 12 in]
        n213 = Unbundle By Name(w793) -> ("V2 Step"=w792:dbl, "V2 Start"=w791:dbl, "Number of points"=w722:i32)
        n214 = Absolute Value(x=w753) -> (abs(x)=w738:dbl[])
        n215 = Absolute Value(x=w755) -> (abs(x)=w754:dbl[])
        n216 = Absolute Value(x=w752) -> (abs(x)=w741:dbl[])
        n217 = Array Size(array=w754) -> (size(s)=w762:i32)
        n218 = Divide(x=w762, y=2) -> (x/y=w705:dbl)
        n219 = Subtract(x=w705, y=1) -> (x-y=w704:dbl)
        n220 = Array Max & Min(array=w738) -> (max value=w745:dbl, min value=w746:dbl)  [unwired: 2 out]
        n221 = Array Max & Min(array=w754) -> (max value=w784:dbl, min value=w751:dbl)  [unwired: 2 out]
        n222 = Array Max & Min(array=w741) -> (max value=w750:dbl, min value=w749:dbl)  [unwired: 2 out]
        n223 = call "4155C Split array.vi"("Number of VAR2 steps"=w722, "Y2 data in"=w755, "X data in"=w786, "Y1 data in"=w753, "Y3 data in"=w752, "error in (no error)"=w775) -> ("Array of clusters"=w777:cluster{"Y data in":dbl[], "X data in":dbl[]}[], "error out"=w710:errorcluster)  [unwired: 1 in]
        n224 = Index Array(array=w738, index=w704) -> (element=w729:dbl)
        n225 = Index Array(array=w738, index=0) -> (element=w730:dbl)
        n226 = Index Array(array=w754, index=w704) -> (element=w731:dbl)
        n227 = Index Array(array=w754, index=0) -> (element=w732:dbl)
        n228 = Index Array(array=w741, index=w704) -> (element=w734:dbl)
        n229 = Index Array(array=w741, index=0) -> (element=w733:dbl)
        n230 = local write "Ig max"(w750) -> ()
        n231 = local write "Ig min"(w749) -> ()
        n232 = local write "Is max"(w745) -> ()
        n233 = local write "Is min"(w746) -> ()
        n234 = local write "Id max"(w784) -> ()
        n235 = local write "Id min"(w751) -> ()
        n236 = local write "I vs Vd"(w777) -> ()
        n237 = Build Array (concatenate)(w744, w745) -> (w723:dbl[])
        n238 = Build Array (concatenate)(w743, w746) -> (w721:dbl[])
        n239 = local write "Is off"(w730) -> ()
        n240 = local write "Is on"(w729) -> ()
        n241 = Build Array (concatenate)(w785, w784) -> (w720:dbl[])
        n242 = Build Array (concatenate)(w772, w751) -> (w719:dbl[])
        n243 = Build Array (concatenate)(w748, w750) -> (w718:dbl[])
        n244 = Build Array (concatenate)(w747, w749) -> (w717:dbl[])
        n245 = Build Array (concatenate)(w736, w729) -> (w716:dbl[])
        n246 = Build Array (concatenate)(w735, w730) -> (w715:dbl[])
        n247 = Build Array (concatenate)(w758, w731) -> (w714:dbl[])
        n248 = Build Array (concatenate)(w759, w732) -> (w713:dbl[])
        n249 = Build Array (concatenate)(w740, w734) -> (w712:dbl[])
        n250 = Build Array (concatenate)(w739, w733) -> (w711:dbl[])
        n251 = local write "Ig off"(w733) -> ()
        n252 = local write "Ig on"(w734) -> ()
        n253 = local write "Id off"(w732) -> ()
        n254 = local write "Id on"(w731) -> ()
        n255 = call "4155C Split array.vi"("Number of VAR2 steps"=w722, "Y2 data in"=w714, "X data in"=w728, "Y1 data in"=w716, "Y3 data in"=w712, "error in (no error)"=w710) -> ("Array of clusters"=w726:cluster{"Y data in":dbl[], "X data in":dbl[]}[], "error out"=w709:errorcluster)  [unwired: 1 in]
        n256 = call "4155C Split array.vi"("Number of VAR2 steps"=w722, "Y2 data in"=w713, "X data in"=w728, "Y1 data in"=w715, "Y3 data in"=w711, "error in (no error)"=w709) -> ("Array of clusters"=w727:cluster{"Y data in":dbl[], "X data in":dbl[]}[], "error out"=w708:errorcluster)  [unwired: 1 in]
        n257 = call "4155C Split array.vi"("Number of VAR2 steps"=w722, "Y2 data in"=w720, "X data in"=w728, "Y1 data in"=w723, "Y3 data in"=w718, "error in (no error)"=w708) -> ("Array of clusters"=w776:cluster{"Y data in":dbl[], "X data in":dbl[]}[], "error out"=w707:errorcluster)  [unwired: 1 in]
        n258 = call "4155C Split array.vi"("Number of VAR2 steps"=w722, "Y2 data in"=w719, "X data in"=w728, "Y1 data in"=w721, "Y3 data in"=w717, "error in (no error)"=w707) -> ("Array of clusters"=w773:cluster{"Y data in":dbl[], "X data in":dbl[]}[], "error out"=w706:errorcluster)  [unwired: 1 in]
        n259 = Open/Create/Replace File(file path (use dialog)=w832, error in=w706, operation (0:open)=w787) -> (refnum out=w770:refnum<file>, error out=w768:errorcluster)  [unwired: 3 in, 1 out]
        n260 = call "4155C Make Big 2d array.vi"("1D Var1"=w786, "1d IS"=w753, "1d ID"=w755, "1d IG"=w752, "1d SMU4"=w790, "SMU4"=w789, "VAR2 START"=w791, "Number of VAR2 steps"=w722, "VAR2 STEP"=w792, "VAR1 Name"="Vd", "Decimal places in header"=i8 1, "VAR2 Name"="Vg") -> ("Header array"=w771:string[], "Data array"=w769:dbl[][])  [unwired: 14 in]
        n261 = local write "Imax vs time"(w776) -> ()
        n262 = local write "Imin vs time"(w773) -> ()
        n263 = local write "Ion vs time"(w726) -> ()
        n264 = local write "Ioff vs time"(w727) -> ()
        n265 = call "4155C Config Chart Colours.vi"("Numeric"=w722, "XY Graph 2"=w757) -> ()  [unwired: 6 in]
        n266 = call "4155C Config Chart Colours.vi"("Numeric"=w722, "XY Graph 2"=w756) -> ()  [unwired: 6 in]
        n267 = call "4155C Config Chart Colours.vi"("Numeric"=w722, "XY Graph 2"=w725) -> ()  [unwired: 6 in]
        n268 = call "4155C Config Chart Colours.vi"("Numeric"=w722, "XY Graph 2"=w724) -> ()  [unwired: 6 in]
        n269 = call "4155C Config Chart Colours.vi"("Numeric"=w722, "XY Graph 2"=w783) -> ()  [unwired: 6 in]
        n270 = call "4155C Write array to file.vi"("Byte Stream File Refnum"=w770, "Header"=w771, "Data Array"=w769, "error in (no error)"=w768) -> ("dup refnum"=w767:refnum<file>, "error out"=w766:errorcluster)  [unwired: 1 in]
        n271 = Close File(refnum=w767, error in=w766) -> (error out=w827:errorcluster)  [unwired: 1 out]
      }
      frame "output-fpp" {
        n272 = Number To Decimal String(number=w854) -> (decimal integer string=w908:string)  [unwired: 1 in]
        n273 = Bundle By Name(cluster=w884, "Emergency Stop"=w911) -> (w921:T2)
        n274 = Delete From Array(array=w899, index=0 ("Index")) -> (deleted portion=w897:string, array with subset deleted=w896:string[])  [unwired: 1 in]
        n275 = VISA Write(VISA resource name=w875, write buffer=":PAGE:CHAN:MODE SWE;" ("write buffer (\"\")"), error in (no error)=w872) -> (VISA resource name out=w874:refnum<visa-resource-name>, error out=w873:errorcluster)  [unwired: 1 out]
        n276 = Concatenate Strings(w907, "-outputfpp-" ("Substring"), w908, w853, ".txt" ("Substring")) -> (w910:string)
        n277 = case shown="\"d\", Default" w897 {
          tunnel: [w922 w923] -> w895
          frame "s" {
            w922 = u16 0 items=["Single", "Double"] ("sweep mode")
          }
          frame "d", Default {
            w923 = u16 1 items=["Single", "Double"] ("sweep mode")
          }
        }
        n278 = Fract/Exp String To Number(string=w896) -> (number=w878:dbl[])  [unwired: 3 in, 1 out]
        n279 = String To Path(string=w910) -> (path=w906:path)
        n280 = Index Array(array=w878, index #1=0 ("Index")) -> (element #1=w894:dbl, element #2=w893:dbl, element #3=w892:dbl)  [unwired: 2 in]
        n281 = Delete From Array(array=w878, length=3 ("Length"), index=0 ("Index")) -> (array with subset deleted=w877:dbl[])  [unwired: 1 out]
        n282 = Bundle By Name(cluster=w886, "Gate Start"=w894, "Gate Stop"=w893, "Gate Step (linear only)"=w892, "Gate Compliance"=w904, "Range mode"=w870, "Range"=w869) -> (w920:T6)
        n283 = Index Array(array=w877, index #1=0 ("Index")) -> (element #1=w889:dbl, element #2=w888:dbl, element #3=w887:dbl)  [unwired: 2 in]
        n284 = call <vilib>:"compatOverwrite.vi"("overwrite (F)"=TRUE) -> ("overwrite?"=w858:T8)
        n285 = Bundle By Name(cluster=w885, "Drain Start"=w889, "Drain Stop"=w888, "Drain Step"=w887, "Drain Compliance"=w905, "Range mode"=w868, "Range"=w871) -> (w919:T7)
        n286 = call "4155C Output-FPP.vi"("VISA resource name in"=w874, "Gate"=w920, "Drain"=w919, "Timings"=w903, "error in (no error)"=w873, "sweep mode"=w895, "Panel controls"=w921) -> ("VD"=w863:dbl[], "Outparams"=w866:T9, "VISA Resource Name out"=w901:refnum<visa-resource-name>, "Vprobe2"=w862:dbl[], "ID"=w861:dbl[], "IG"=w860:dbl[], "Vprobe1"=w859:dbl[], "error out"=w902:errorcluster)  [unwired: 13 in]
        n287 = Unbundle By Name(w866) -> ("V2 Step"=w867:dbl, "V2 Start"=w865:dbl, "Number of points"=w864:i32)
        n288 = Open/Create/Replace File(file path (use dialog)=w906, error in=w902, operation (0:open)=w858) -> (refnum out=w916:refnum<file>, error out=w917:errorcluster)  [unwired: 3 in, 1 out]
        n289 = call "4155C Make Big 2d array FPP.vi"("1D Var1"=w863, "1d ID"=w861, "1d Vp2"=w862, "1d IG"=w860, "1d Vp1"=w859, "VAR2 START"=w865, "Number of VAR2 steps"=w864, "VAR2 STEP"=w867, "VAR1 Name"="Vd", "Decimal places in header"=i8 1, "VAR2 Name"="Vg") -> ("Header array"=w912:string[], "Data array"=w913:dbl[][])  [unwired: 15 in]
        n290 = call "4155C Write array to file.vi"("Byte Stream File Refnum"=w916, "Header"=w912, "Data Array"=w913, "error in (no error)"=w917) -> ("dup refnum"=w914:refnum<file>, "error out"=w915:errorcluster)  [unwired: 1 in]
        n291 = Close File(refnum=w914, error in=w915) -> (error out=w900:errorcluster)  [unwired: 1 out]
      }
      frame "itime" {
        n292 = Delete From Array(array=w926, index=1) -> (deleted portion=w925:string)  [unwired: 1 in, 1 out]
        n293 = Delete From Array(array=w926, index=0 ("Index")) -> (deleted portion=w955:string)  [unwired: 1 in, 1 out]
        n294 = Fract/Exp String To Number(string=w925) -> (number=w924:dbl)  [unwired: 3 in, 1 out]
        n295 = case shown="\"l\"" w955 {
          tunnel: w954 -> [w960 w962 w966]
          tunnel: [w959 w961 w965] -> w947
          tunnel: w924 -> [w957 _ w964]
          frame "s" {
            w958 = u32 0 items=["short  ", "medium  ", "long  "] ("integration time 2")
            n296 = Bundle By Name(cluster=w960, "integration time"=w958, "Short/Long integration time"=w957) -> (w959:T5)
          }
          frame "m", Default {
            w963 = u32 1 items=["short  ", "medium  ", "long  "] ("integration time 2")
            n297 = Bundle By Name(cluster=w962, "integration time"=w963) -> (w961:T5)
          }
          frame "l" {
            w967 = u32 2 items=["short  ", "medium  ", "long  "] ("integration time 2")
            n298 = Bundle By Name(cluster=w966, "integration time"=w967, "Short/Long integration time"=w964) -> (w965:T5)
          }
        }
      }
      frame "pulsed" {
        n299 = Delete From Array(array=w996, index=0 ("Index")) -> (deleted portion=w997:string, array with subset deleted=w984:string[])  [unwired: 1 in]
        n300 = case shown="\"on\", Default" w997 {
          tunnel: w995 -> [w1007 w1010]
          tunnel: [w1006 w1009] -> w988
          tunnel: w984 -> [w1004 _]
          frame "on", Default {
            w1005 = u16 1 items=["Continuous", "Pulsed"] ("sweep method")
            n301 = Fract/Exp String To Number(string=w1004) -> (number=w1002:dbl[])  [unwired: 3 in, 1 out]
            n302 = Index Array(array=w1002, index #1=0 ("Index")) -> (element #1=w1001:dbl, element #2=w1000:dbl, element #3=w999:dbl)  [unwired: 2 in]
            n303 = Bundle By Name(cluster=w1007, "sweep method"=w1005, "Pulse period"=w1001, "Base voltage"=w1000, "Pulse width"=w999) -> (w1006:T5)
          }
          frame "off" {
            w1008 = u16 0 items=["Continuous", "Pulsed"] ("sweep method")
            n304 = Bundle By Name(cluster=w1010, "sweep method"=w1008) -> (w1009:T5)
          }
        }
      }
      frame "gaterangemode" {
        n305 = Delete From Array(array=w1037, index=0 ("Index")) -> (deleted portion=w1038:string)  [unwired: 1 in, 1 out]
        n306 = case shown="\"f\"" w1038 {
          tunnel: [w1040 w1041 w1042] -> w1027
          frame "a", Default {
            w1040 = u16 0 items=["Auto", "Limited", "Fixed"] ("Gate Range\nmode 2")
          }
          frame "f" {
            w1041 = u16 2 items=["Auto", "Limited", "Fixed"] ("Gate Range\nmode 2")
          }
          frame "l" {
            w1042 = u16 1 items=["Auto", "Limited", "Fixed"] ("Gate Range\nmode 2")
          }
        }
      }
      frame "gaterange" {
        (unwired) u8 11 items=["10fA  ", "100fA  ", "1nA  ", "10nA", "100nA", "1uA", "10uA", "100uA", "1mA", "10mA", "100mA", "1A"] ("Gate Range 2")
        n307 = Delete From Array(array=w1076, index=0 ("Index")) -> (deleted portion=w1066:string)  [unwired: 1 in, 1 out]
        n308 = Scan Value(string=w1066, format string="") -> (value=w1064:dbl)  [unwired: 1 in, 1 out]
        n309 = Logarithm Base 10(1:w1064) -> (0:w1063:dbl)
        n310 = Round To Nearest(number=w1063) -> (nearest integer value=w1062:dbl)
        n311 = Add(x=w1062, y=11.0) -> (x+y=w1060:dbl)
        n312 = To Unsigned Byte Integer(number=w1060) -> (unsigned 8bit integer=w1059:u8)
      }
      frame "drainrange" {
        (unwired) u8 11 items=["10fA  ", "100fA  ", "1nA  ", "10nA", "100nA", "1uA", "10uA", "100uA", "1mA", "10mA", "100mA", "1A"] ("Gate Range 2")
        n313 = Delete From Array(array=w1111, index=0 ("Index")) -> (deleted portion=w1102:string)  [unwired: 1 in, 1 out]
        n314 = Scan Value(string=w1102, format string="") -> (value=w1100:dbl)  [unwired: 1 in, 1 out]
        n315 = Logarithm Base 10(1:w1100) -> (0:w1099:dbl)
        n316 = Round To Nearest(number=w1099) -> (nearest integer value=w1098:dbl)
        n317 = Add(x=w1098, y=11.0) -> (x+y=w1096:dbl)
        n318 = To Unsigned Byte Integer(number=w1096) -> (unsigned 8bit integer=w1095:u8)
      }
      frame "drainrangemode" {
        n319 = Delete From Array(array=w1139, index=0 ("Index")) -> (deleted portion=w1140:string)  [unwired: 1 in, 1 out]
        n320 = case shown="\"f\"" w1140 {
          tunnel: [w1142 w1143 w1144] -> w1129
          frame "a", Default {
            w1142 = u16 0 items=["Auto", "Limited", "Fixed"] ("Gate Range\nmode 2")
          }
          frame "f" {
            w1143 = u16 2 items=["Auto", "Limited", "Fixed"] ("Gate Range\nmode 2")
          }
          frame "l" {
            w1144 = u16 1 items=["Auto", "Limited", "Fixed"] ("Gate Range\nmode 2")
          }
        }
      }
      frame "Error", Default {
      }
      frame "logfile" {
        n321 = Number To Decimal String(number=w1187) -> (decimal integer string=w1222:string)  [unwired: 1 in]
        n322 = Concatenate Strings(w1221, "logfile" ("Substring"), w1222, w1185, ".txt" ("Substring")) -> (w1219:string)
        n323 = String To Path(string=w1219) -> (path=w1192:path)
        n324 = Unbundle(w1218) -> ("integration time"=w1217:u32, "Short/Long integration time"=w1216:dbl, "hold time (sec)"=w1215:dbl, "delay time (sec)"=w1214:dbl, "Step Time (0 disables)"=w1213:dbl, "sweep method"=w1212:u16, "Pulse period"=w1211:dbl, "Base voltage"=w1210:dbl, "Pulse width"=w1209:dbl)
        n325 = Build Array(w1217, w1216, w1215, w1214, w1213, w1212, w1211, w1210, w1209, w1203, w1204, w1205, w1206, w1207, w1208) -> (w1196:dbl[])
        n326 = Insert Into Array(array=dbl[][] [] ("Input Array"), new element=w1196) -> (w1195:dbl[][])  [unwired: 2 in]
        n327 = call <vilib>:"compatOverwrite.vi"("overwrite (F)"=TRUE) -> ("overwrite?"=w1190:T8)
        n328 = Open/Create/Replace File(file path (use dialog)=w1192, error in=w1194, operation (0:open)=w1190) -> (refnum out=w1200:refnum<file>, error out=w1199:errorcluster)  [unwired: 3 in, 1 out]
        n329 = call "4155C Write array to file.vi"("Byte Stream File Refnum"=w1200, "Header"=string[] ["Int Time", "Short/Long Itime", "Hold time", "Delay time", "Step time", "Sweep method", "Pulse period", "Base Voltage", "Pulse width", "Drain compliance", "Gate compliance", "Gate range mode", "Gate range", "S/D range mode", "S/D range"], "Data Array"=w1195, "error in (no error)"=w1199) -> ("dup refnum"=w1202:refnum<file>, "error out"=w1201:errorcluster)  [unwired: 1 in]
        n330 = Close File(refnum=w1202, error in=w1201) -> (error out=w1193:errorcluster)  [unwired: 1 out]
      }
      frame "sample" {
        n331 = Number To Decimal String(number=w1240) -> (decimal integer string=w1288:string)  [unwired: 1 in]
        n332 = Fract/Exp String To Number(string=w1285) -> (number=w1246:dbl[])  [unwired: 3 in, 1 out]
        n333 = Concatenate Strings(w1263, "-sample-" ("Substring"), w1288, w1238, ".txt" ("Substring")) -> (w1286:string)
        n334 = Index Array(array=w1246, index=0 ("Index")) -> (element=w1283:dbl)
        n335 = String To Path(string=w1286) -> (path=w1267:path)
        n336 = Index Array(array=w1246, index=2 ("Index")) -> (element=w1279:dbl)
        n337 = Index Array(array=w1246, index=3 ("Index")) -> (element=w1248:dbl)
        n338 = Index Array(array=w1246, index=4 ("Index")) -> (element=w1245:dbl)
        n339 = call "4155C Config Sampling Measurements.vi"("Sampling interval"=w1245, "Sample time"=w1248, "Display on/off"=TRUE, "Timings"=w1254, "Num Points"=w1279, "error in (no error)"=w1290, "Drain Compliance"=w1289, "Gate Compliance"=w1264, "VISA session"=w1291) -> ("error out"=w1292:errorcluster, "dup VISA resource name"=w1293:refnum<visa-resource-name>)  [unwired: 1 in]
        n340 = Index Array(array=w1246, index=1 ("Index")) -> (element=w1280:dbl)
        n341 = call "4155C Take Sample.vi"("Emergency Stop"=w1260, "error in (no error)"=w1292, "Vd"=w1280, "Vg"=w1283, "VISA resource name in"=w1293) -> ("error out"=w1258:errorcluster, "Id"=w1295:dbl[], "Ig"=w1269:dbl[], "VISA Resource Name out"=w1256:refnum<visa-resource-name>, "Is"=w1294:dbl[], "Time"=w1273:dbl[])  [unwired: 1 in]
        n342 = Insert Into Array(array=dbl[][] [] ("Input Array"), new element=w1273) -> (w1272:dbl[][])  [unwired: 2 in]
        n343 = Insert Into Array(array=w1272, new element=w1269) -> (w1271:dbl[][])  [unwired: 2 in]
        n344 = Insert Into Array(array=w1271, new element=w1295) -> (w1270:dbl[][])  [unwired: 2 in]
        n345 = VISA Write(VISA resource name=w1256, write buffer=":DISP ON" ("write buffer (\"\")"), error in (no error)=w1258) -> (VISA resource name out=w1255:refnum<visa-resource-name>, error out=w1257:errorcluster)  [unwired: 1 out]
        n346 = Insert Into Array(array=w1270, new element=w1294) -> (w1262:dbl[][])  [unwired: 2 in]
        n347 = Transpose 2D Array(2D array=w1262) -> (transposed array=w1261:dbl[][])
        n348 = call <vilib>:"compatOverwrite.vi"("overwrite (F)"=TRUE) -> ("overwrite?"=w1243:T8)
        n349 = Open/Create/Replace File(file path (use dialog)=w1267, error in=w1257, operation (0:open)=w1243) -> (refnum out=w1276:refnum<file>, error out=w1275:errorcluster)  [unwired: 3 in, 1 out]
        n350 = call "4155C Write array to file.vi"("Byte Stream File Refnum"=w1276, "Header"=string[] ["Time /s", "Ig /A", "Id /A", "Is /A"], "Data Array"=w1261, "error in (no error)"=w1275) -> ("dup refnum"=w1278:refnum<file>, "error out"=w1277:errorcluster)  [unwired: 1 in]
        n351 = Close File(refnum=w1278, error in=w1277) -> (error out=w1265:errorcluster)  [unwired: 1 out]
      }
      frame "samplei" {
        n352 = Number To Decimal String(number=w1312) -> (decimal integer string=w1363:string)  [unwired: 1 in]
        n353 = Concatenate Strings(w1342, "-samplei-" ("Substring"), w1363, w1311, ".txt" ("Substring")) -> (w1361:string)
        n354 = Fract/Exp String To Number(string=w1360) -> (number=w1327:dbl[])  [unwired: 3 in, 1 out]
        n355 = String To Path(string=w1361) -> (path=w1345:path)
        n356 = Index Array(array=w1327, index=4 ("Index")) -> (element=w1321:dbl)
        n357 = Index Array(array=w1327, index=3 ("Index")) -> (element=w1322:dbl)
        n358 = Index Array(array=w1327, index=1 ("Index")) -> (element=w1324:dbl)
        n359 = Index Array(array=w1327, index=0 ("Index")) -> (element=w1325:dbl)
        n360 = Index Array(array=w1327, index=2 ("Index")) -> (element=w1323:dbl)
        n361 = call "4155C Config SamplingI Measurements.vi"("Sample time"=w1323, "Display on/off"=TRUE, "Timings"=w1334, "Num Points"=w1324, "error in (no error)"=w1365, "Sampling interval"=w1322, "VISA session"=w1366) -> ("error out"=w1367:errorcluster, "dup VISA resource name"=w1368:refnum<visa-resource-name>)  [unwired: 3 in]
        n362 = call "4155C Take SampleI.vi"("Emergency Stop"=w1339, "error in (no error)"=w1367, "Idg 2"=w1325, "Vdg compliance 2"=w1321, "VISA resource name in"=w1368) -> ("error out"=w1337:errorcluster, "Idg"=w1370:dbl[], "Vdg"=w1347:dbl[], "VISA Resource Name out"=w1335:refnum<visa-resource-name>, "Is"=w1369:dbl[], "Time"=w1351:dbl[])  [unwired: 1 in]
        n363 = Insert Into Array(array=dbl[][] [] ("Input Array"), new element=w1351) -> (w1350:dbl[][])  [unwired: 2 in]
        n364 = Insert Into Array(array=w1350, new element=w1347) -> (w1349:dbl[][])  [unwired: 2 in]
        n365 = Insert Into Array(array=w1349, new element=w1370) -> (w1348:dbl[][])  [unwired: 2 in]
        n366 = VISA Write(VISA resource name=w1335, write buffer=":DISP ON" ("write buffer (\"\")"), error in (no error)=w1337) -> (VISA resource name out=w1320:refnum<visa-resource-name>, error out=w1336:errorcluster)  [unwired: 1 out]
        n367 = Insert Into Array(array=w1348, new element=w1369) -> (w1341:dbl[][])  [unwired: 2 in]
        n368 = call <vilib>:"compatOverwrite.vi"("overwrite (F)"=TRUE) -> ("overwrite?"=w1315:T8)
        n369 = Open/Create/Replace File(file path (use dialog)=w1345, error in=w1336, operation (0:open)=w1315) -> (refnum out=w1354:refnum<file>, error out=w1353:errorcluster)  [unwired: 3 in, 1 out]
        n370 = Transpose 2D Array(2D array=w1341) -> (transposed array=w1340:dbl[][])
        n371 = call "4155C Write array to file.vi"("Byte Stream File Refnum"=w1354, "Header"=string[] ["Time /s", "Vdg /V", "Idg /A", "Is /A"], "Data Array"=w1340, "error in (no error)"=w1353) -> ("dup refnum"=w1356:refnum<file>, "error out"=w1355:errorcluster)  [unwired: 1 in]
        n372 = Close File(refnum=w1356, error in=w1355) -> (error out=w1318:errorcluster)  [unwired: 1 out]
        n373 = VISA Write(VISA resource name=w1320, write buffer=";:PAGE:SCON:STAN OFF;:PAGE:CHAN:VSU2:DIS;" ("write buffer (\"\")"), error in (no error)=w1318) -> (VISA resource name out=w1316:refnum<visa-resource-name>, error out=w1317:errorcluster)  [unwired: 1 out]
      }
      frame "#" {
        n374 = VISA Write(VISA resource name=w1391, write buffer=":DISP ON" ("write buffer (\"\")"), error in (no error)=w1390) -> (VISA resource name out=w1389:refnum<visa-resource-name>, error out=w1388:errorcluster)  [unwired: 1 out]
      }
      frame "stressV" {
        n375 = Number To Decimal String(number=w1415) -> (decimal integer string=w1456:string)  [unwired: 1 in]
        n376 = Concatenate Strings(w1440, "-stressV-" ("Substring"), w1456, w1414, ".txt" ("Substring")) -> (w1454:string)
        n377 = Fract/Exp String To Number(string=w1453) -> (number=w1426:dbl[])  [unwired: 3 in, 1 out]
        n378 = String To Path(string=w1454) -> (path=w1444:path)
        n379 = Index Array(array=w1426, index=3 ("Index")) -> (element=w1423:dbl)
        n380 = Index Array(array=w1426, index=1 ("Index")) -> (element=w1421:dbl)
        n381 = Index Array(array=w1426, index=0 ("Index")) -> (element=w1420:dbl)
        n382 = Index Array(array=w1426, index=4 ("Index")) -> (element=w1425:dbl)
        n383 = Index Array(array=w1426, index=2 ("Index")) -> (element=w1422:dbl)
        n384 = call "4155C Config V Stress.vi"("VISA session"=w1459, "ID compliance"=w1423, "VD"=w1421, "VG"=w1420, "IG compliance"=w1422, "error in (no error)"=w1458, "Display on/off"=TRUE) -> ("dup VISA resource name"=w1461:refnum<visa-resource-name>, "error out"=w1460:errorcluster)
        n385 = call "4155C Apply Stress.vi"("error in (no error)"=w1460, "Duration"=w1425, "Emergency Stop"=w1439, "VISA resource name in"=w1461) -> ("error out"=w1437:errorcluster, "VISA Resource Name out"=w1435:refnum<visa-resource-name>)
        n386 = VISA Write(VISA resource name=w1435, write buffer=":DISP ON" ("write buffer (\"\")"), error in (no error)=w1437) -> (VISA resource name out=w1434:refnum<visa-resource-name>, error out=w1436:errorcluster)  [unwired: 1 out]
        n387 = call <vilib>:"compatOverwrite.vi"("overwrite (F)"=TRUE) -> ("overwrite?"=w1419:T8)
        n388 = Open/Create/Replace File(file path (use dialog)=w1444, error in=w1436, operation (0:open)=w1419) -> (refnum out=w1447:refnum<file>, error out=w1446:errorcluster)  [unwired: 3 in, 1 out]
        n389 = call "4155C Write array to file.vi"("Byte Stream File Refnum"=w1447, "Header"=string[] ["V stress completed successfully", ""], "error in (no error)"=w1446) -> ("dup refnum"=w1449:refnum<file>, "error out"=w1448:errorcluster)  [unwired: 2 in]
        n390 = Close File(refnum=w1449, error in=w1448) -> (error out=w1442:errorcluster)  [unwired: 1 out]
      }
      frame "stressI" {
        n391 = Number To Decimal String(number=w1477) -> (decimal integer string=w1514:string)  [unwired: 1 in]
        n392 = Concatenate Strings(w1498, "-stressI-" ("Substring"), w1514, w1476, ".txt" ("Substring")) -> (w1512:string)
        n393 = Fract/Exp String To Number(string=w1511) -> (number=w1486:dbl[])  [unwired: 3 in, 1 out]
        n394 = Index Array(array=w1486, index=1 ("Index")) -> (element=w1482:dbl)
        n395 = Index Array(array=w1486, index=0 ("Index")) -> (element=w1483:dbl)
        n396 = call "4155C Config I Stress.vi"("VISA session"=w1517, "IDG"=w1483, "VDG compliance"=w1482, "error in (no error)"=w1516, "Display on/off"=TRUE) -> ("dup VISA resource name"=w1519:refnum<visa-resource-name>, "error out"=w1518:errorcluster)
        n397 = Index Array(array=w1486, index=2 ("Index")) -> (element=w1484:dbl)
        n398 = String To Path(string=w1512) -> (path=w1502:path)
        n399 = call "4155C Apply Stress.vi"("error in (no error)"=w1518, "Duration"=w1484, "Emergency Stop"=w1497, "VISA resource name in"=w1519) -> ("error out"=w1495:errorcluster, "VISA Resource Name out"=w1493:refnum<visa-resource-name>)
        n400 = VISA Write(VISA resource name=w1493, write buffer=":DISP ON" ("write buffer (\"\")"), error in (no error)=w1495) -> (VISA resource name out=w1492:refnum<visa-resource-name>, error out=w1494:errorcluster)  [unwired: 1 out]
        n401 = call <vilib>:"compatOverwrite.vi"("overwrite (F)"=TRUE) -> ("overwrite?"=w1481:T8)
        n402 = Open/Create/Replace File(file path (use dialog)=w1502, error in=w1494, operation (0:open)=w1481) -> (refnum out=w1505:refnum<file>, error out=w1504:errorcluster)  [unwired: 3 in, 1 out]
        n403 = call "4155C Write array to file.vi"("Byte Stream File Refnum"=w1505, "Header"=string[] ["I stress completed successfully", ""], "error in (no error)"=w1504) -> ("dup refnum"=w1507:refnum<file>, "error out"=w1506:errorcluster)  [unwired: 2 in]
        n404 = Close File(refnum=w1507, error in=w1506) -> (error out=w1500:errorcluster)  [unwired: 1 out]
      }
      frame "vsu2pulse" {
        n405 = Number To Decimal String(number=w1535) -> (decimal integer string=w1570:string)  [unwired: 1 in]
        n406 = Concatenate Strings(w1555, "-vsu2-" ("Substring"), w1570, w1534, ".txt" ("Substring")) -> (w1568:string)
        n407 = Fract/Exp String To Number(string=w1567) -> (number=w1543:dbl[])  [unwired: 3 in, 1 out]
        n408 = String To Path(string=w1568) -> (path=w1559:path)
        n409 = Index Array(array=w1543, index=1 ("Index")) -> (element=w1542:dbl)
        n410 = Index Array(array=w1543, index=0 ("Index")) -> (element=w1540:dbl)
        n411 = call "4155C Config VSU2 Stress.vi"("error in (no error)"=w1572, "VSU2"=w1540, "Display on/off"=TRUE, "VISA session"=w1573) -> ("error out"=w1574:errorcluster, "dup VISA resource name"=w1575:refnum<visa-resource-name>)
        n412 = call "4155C Apply Stress.vi"("error in (no error)"=w1574, "Duration"=w1542, "Emergency Stop"=w1554, "VISA resource name in"=w1575) -> ("error out"=w1552:errorcluster, "VISA Resource Name out"=w1550:refnum<visa-resource-name>)
        n413 = VISA Write(VISA resource name=w1550, write buffer=":DISP ON" ("write buffer (\"\")"), error in (no error)=w1552) -> (VISA resource name out=w1549:refnum<visa-resource-name>, error out=w1551:errorcluster)  [unwired: 1 out]
        n414 = call <vilib>:"compatOverwrite.vi"("overwrite (F)"=TRUE) -> ("overwrite?"=w1539:T8)
        n415 = Open/Create/Replace File(file path (use dialog)=w1559, error in=w1551, operation (0:open)=w1539) -> (refnum out=w1562:refnum<file>, error out=w1561:errorcluster)  [unwired: 3 in, 1 out]
        n416 = call "4155C Write array to file.vi"("Byte Stream File Refnum"=w1562, "Header"=string[] ["VSU2 pulse completed successfully", ""], "error in (no error)"=w1561) -> ("dup refnum"=w1564:refnum<file>, "error out"=w1563:errorcluster)  [unwired: 2 in]
        n417 = Close File(refnum=w1564, error in=w1563) -> (error out=w1557:errorcluster)  [unwired: 1 out]
      }
      frame "sample-fpp" {
        w1602 = string[] ["Time /s", "Id VgVd /A", "Ig VgVd /A", "Vp1 VgVd /V", "Vp2 VgVd /V"] ("Header")
        w1606 = "%d" ("format string")
        n418 = Number To Decimal String(number=w1591) -> (decimal integer string=w1654:string)  [unwired: 1 in]
        n419 = Fract/Exp String To Number(string=w1651) -> (number=w1639:dbl[])  [unwired: 3 in, 1 out]
        n420 = Concatenate Strings(w1645, "-samplefpp-" ("Substring"), w1654, w1590, ".txt" ("Substring")) -> (w1652:string)
        n421 = String To Path(string=w1652) -> (path=w1614:path)
        n422 = Index Array(array=w1639, index=0 ("Index")) -> (element=w1600:dbl)
        n423 = Index Array(array=w1639, index=1 ("Index")) -> (element=w1599:dbl)
        n424 = Index Array(array=w1639, index=2 ("Index")) -> (element=w1647:dbl)
        n425 = Index Array(array=w1639, index=3 ("Index")) -> (element=w1637:dbl)
        n426 = call "4155C Config Sampling Measurements FPP.vi"("VISA session"=w1657, "Num Points"=w1647, "Vg"=w1600, "Display on/off"=TRUE, "Gate Compliance"=w1646, "Drain Compliance"=w1655, "Standby"="Standby", "error in (no error)"=w1656, "Timings"=w1644, "Vd"=w1599, "Sample time"=w1637) -> ("dup VISA resource name"=w1616:refnum<visa-resource-name>, "error out"=w1615:errorcluster)  [unwired: 3 in]
        n427 = Number To Decimal String(number=w1600) -> (decimal integer string=w1626:string)  [unwired: 1 in]
        n428 = call "4155C Take Sample FPP.vi"("VISA resource name in"=w1616, "error in (no error)"=w1615, "Emergency Stop"=w1617) -> ("Time"=w1621:dbl[], "Vp1"=w1631:dbl[], "VISA Resource Name out"=w1597:refnum<visa-resource-name>, "Ig"=w1619:dbl[], "Id"=w1620:dbl[], "Vp2"=w1629:dbl[], "error out"=w1618:errorcluster)  [unwired: 10 in]
        n429 = Insert Into Array(array=dbl[][] [] ("Input Array"), new element=w1621) -> (w1635:dbl[][])  [unwired: 2 in]
        n430 = Number To Decimal String(number=w1599) -> (decimal integer string=w1624:string)  [unwired: 1 in]
        n431 = Insert Into Array(array=w1635, new element=w1620) -> (w1634:dbl[][])  [unwired: 2 in]
        n432 = Concatenate Strings("(Vg = " ("Substring"), w1626, "V, Vd = " ("Substring"), w1624, "V)" ("Substring")) -> (w1622:string)
        n433 = Insert Into Array(array=w1634, new element=w1619) -> (w1633:dbl[][])  [unwired: 2 in]
        n434 = Insert Into Array(array=w1633, new element=w1631) -> (w1630:dbl[][])  [unwired: 2 in]
        n435 = Insert Into Array(array=w1630, new element=w1629) -> (w1598:dbl[][])  [unwired: 2 in]
        n436 = Transpose 2D Array(2D array=w1598) -> (transposed array=w1628:dbl[][])
        n437 = call <vilib>:"compatOverwrite.vi"("overwrite (F)"=TRUE) -> ("overwrite?"=w1595:T8)
        n438 = Open/Create/Replace File(file path (use dialog)=w1614, error in=w1618, operation (0:open)=w1595) -> (refnum out=w1611:refnum<file>, error out=w1612:errorcluster)  [unwired: 3 in, 1 out]
        n439 = Array To Spreadsheet String(array=w1602, 3:w1606) -> (spreadsheet string=w1608:string)  [unwired: 1 in]
        n440 = Search and Replace String(replace all?=TRUE ("replace all? (F)"), input string=w1608, search string="VgVd", replace string=w1622) -> (result string=w1604:string)  [unwired: 4 in, 3 out]
        n441 = Spreadsheet String To Array(format string=w1606, spreadsheet string=w1604, array type (2D Dbl)=w1602) -> (array=w1603:string[])  [unwired: 1 in]
        n442 = call "4155C Write array to file.vi"("Byte Stream File Refnum"=w1611, "Header"=w1603, "Data Array"=w1628, "error in (no error)"=w1612) -> ("dup refnum"=w1609:refnum<file>, "error out"=w1610:errorcluster)  [unwired: 1 in]
        n443 = Close File(refnum=w1609, error in=w1610) -> (error out=w1596:errorcluster)  [unwired: 1 out]
      }
      frame "resample-fpp" {
        w1686 = string[] ["Time /s", "Id VgVd /A", "Ig VgVd /A", "Vp1 VgVd /V", "Vp2 VgVd /V"] ("Header")
        w1690 = "%d" ("format string")
        n444 = Number To Decimal String(number=w1672) -> (decimal integer string=w1730:string)  [unwired: 1 in]
        n445 = Fract/Exp String To Number(string=w1727) -> (number=w1679:dbl[])  [unwired: 3 in, 1 out]
        n446 = Concatenate Strings(w1723, "-resamplefpp-" ("Substring"), w1730, w1673, ".txt" ("Substring")) -> (w1728:string)
        n447 = String To Path(string=w1728) -> (path=w1698:path)
        n448 = Index Array(array=w1679, index=0 ("Index")) -> (element=w1685:dbl)
        n449 = Index Array(array=w1679, index=1 ("Index")) -> (element=w1684:dbl)
        n450 = Number To Decimal String(number=w1685) -> (decimal integer string=w1708:string)  [unwired: 1 in]
        n451 = call "4155C Take Sample FPP.vi"("VISA resource name in"=w1681, "error in (no error)"=w1680, "Emergency Stop"=w1699) -> ("Time"=w1703:dbl[], "Vp1"=w1713:dbl[], "VISA Resource Name out"=w1683:refnum<visa-resource-name>, "Ig"=w1701:dbl[], "Id"=w1702:dbl[], "Vp2"=w1711:dbl[], "error out"=w1700:errorcluster)  [unwired: 10 in]
        n452 = Insert Into Array(array=dbl[][] [] ("Input Array"), new element=w1703) -> (w1717:dbl[][])  [unwired: 2 in]
        n453 = Number To Decimal String(number=w1684) -> (decimal integer string=w1706:string)  [unwired: 1 in]
        n454 = Insert Into Array(array=w1717, new element=w1702) -> (w1716:dbl[][])  [unwired: 2 in]
        n455 = Concatenate Strings("(Vg = " ("Substring"), w1708, "V, Vd = " ("Substring"), w1706, "V)" ("Substring")) -> (w1704:string)
        n456 = Insert Into Array(array=w1716, new element=w1701) -> (w1715:dbl[][])  [unwired: 2 in]
        n457 = Insert Into Array(array=w1715, new element=w1713) -> (w1712:dbl[][])  [unwired: 2 in]
        n458 = Insert Into Array(array=w1712, new element=w1711) -> (w1678:dbl[][])  [unwired: 2 in]
        n459 = call <vilib>:"compatOverwrite.vi"("overwrite (F)"=TRUE) -> ("overwrite?"=w1677:T8)
        n460 = Open/Create/Replace File(file path (use dialog)=w1698, error in=w1700, operation (0:open)=w1677) -> (refnum out=w1695:refnum<file>, error out=w1696:errorcluster)  [unwired: 3 in, 1 out]
        n461 = Array To Spreadsheet String(array=w1686, 3:w1690) -> (spreadsheet string=w1692:string)  [unwired: 1 in]
        n462 = Transpose 2D Array(2D array=w1678) -> (transposed array=w1710:dbl[][])
        n463 = Search and Replace String(replace all?=TRUE ("replace all? (F)"), input string=w1692, search string="VgVd", replace string=w1704) -> (result string=w1688:string)  [unwired: 4 in, 3 out]
        n464 = Spreadsheet String To Array(format string=w1690, spreadsheet string=w1688, array type (2D Dbl)=w1686) -> (array=w1687:string[])  [unwired: 1 in]
        n465 = call "4155C Write array to file.vi"("Byte Stream File Refnum"=w1695, "Header"=w1687, "Data Array"=w1710, "error in (no error)"=w1696) -> ("dup refnum"=w1693:refnum<file>, "error out"=w1694:errorcluster)  [unwired: 1 in]
        n466 = Close File(refnum=w1693, error in=w1694) -> (error out=w1682:errorcluster)  [unwired: 1 out]
      }
      frame "serial" {
        n467 = local read "Termination char\n(0xA = '\\n' = LF)\n(0xD = '\\r' = CR)"() -> (w1753:u8)
        n468 = local read "Enable Termination\nChar (T)"() -> (w1754:bool)
        n469 = Index Array(array=w1761, index=0 ("Index")) -> (element=w1760:string)
        n470 = local read "parity"() -> (w1744:u16)
        n471 = local read "Delay before read (ms)"() -> (w1755:u32)
        n472 = local read "byte count"() -> (w1752:u32)
        n473 = local read "Timeout (ms)"() -> (w1751:u32)
        n474 = local read "VISA resource name"() -> (w1748:refnum<visa-resource-name>)
        n475 = local read "baud rate"() -> (w1747:u32)
        n476 = local read "Serial End Mode for Reads"() -> (w1746:u16)
        n477 = local read "data bits"() -> (w1745:u16)
        n478 = local read "stop bits"() -> (w1750:u16)
        n479 = local read "flow control"() -> (w1749:u16)
        n480 = call "Serial write and read v0.5.vi"("Delay before read (ms)"=w1755, "Termination char\n(0xA = '\\n' = LF)\n(0xD = '\\r' = CR)"=w1753, "Enable Termination\nChar (T)"=w1754, "parity"=w1744, "stop bits"=w1750, "string to write"=w1760, "flow control"=w1749, "byte count"=w1752, "Serial Settings:Serial End Mode for Reads"=w1746, "Timeout (ms)"=w1751, "error in (no error)"=w1766, "VISA resource name"=w1748, "baud rate"=w1747, "data bits"=w1745) -> ("Serial port output"=w1756:string, "error out"=w1765:errorcluster)
        n481 = Build Array (concatenate)(w1756, w1757) -> (w1758:string[])
      }
    }
    n482 = local read "Time Units"() -> (w65:u16)
    n483 = case shown="0" w65 {
      tunnel: ["Time (Seconds)" ("element") "Time (Minutes)" ("element") "Time (Hours)" ("element")] -> w105
      frame 0 {
      }
      frame 1, Default {
      }
      frame 2 {
      }
    }
    n484 = Build Array(w118, w73, w83, w82, w81, w80, w79, w78, w77, w76, w75, w74, w72) -> (w142:dbl[][])
    n485 = Transpose 2D Array(2D array=w142) -> (transposed array=w141:dbl[][])
    n486 = Concatenate Strings(w70, "-Imax_Imin_Ion_Ioff_vs_time.txt" ("Suffix (Imax,Imin,Ion,Ioff)")) -> (w152:string)
    n487 = Build Array(w105, "Is max (A)" ("VAR2 Name"), "Is min (A)" ("VAR2 Name"), "Id max (A)" ("VAR2 Name"), "Id min (A)" ("VAR2 Name"), "Ig max (A)" ("VAR2 Name"), "Ig min (A)" ("VAR2 Name"), "Is on (A)" ("VAR2 Name"), "Is off (A)" ("VAR2 Name"), "Id on (A)" ("VAR2 Name"), "Id off (A)" ("VAR2 Name"), "Ig on (A)" ("VAR2 Name"), "Ig off (A)" ("VAR2 Name")) -> (w147:string[])
    n488 = Array To Spreadsheet String(array=w141, 3:"%e" ("format string")) -> (spreadsheet string=w145:string)  [unwired: 1 in]
    n489 = Array To Spreadsheet String(array=w147, 3:"" ("format string")) -> (spreadsheet string=w146:string)  [unwired: 1 in]
    n490 = String To Path(string=w152) -> (path=w151:path)
    n491 = Build Array(w146, w145) -> (w144:string[])
    n492 = Write to Text File(file (use dialog)=w151, text=w144, error in=w116) -> (refnum out=w153:refnum<file>, error out=w143:errorcluster)  [unwired: 1 in, 1 out]
    n493 = Close File(refnum=w153, error in=w143) -> (error out=w69:errorcluster)  [unwired: 1 out]
    n494 = Concatenate Strings(w70, "-serial_port_output.txt" ("Suffix (serial port log)")) -> (w122:string)
    n495 = String To Path(string=w122) -> (path=w121:path)
    n496 = Build Array(w105, "Serial port input" ("VAR2 Name"), "Serial port output: ") -> (w109:string[])
    n497 = Array To Spreadsheet String(array=w113, 3:"" ("format string")) -> (spreadsheet string=w106:string)  [unwired: 1 in]
    n498 = Array To Spreadsheet String(array=w109, 3:"" ("format string")) -> (spreadsheet string=w107:string)  [unwired: 1 in]
    n499 = Build Array(w107, w106) -> (w108:string[])
    n500 = Array To Spreadsheet String(array=w112, 3:"" ("format string")) -> (spreadsheet string=w127:string)  [unwired: 1 in]
    n501 = Write to Text File(file (use dialog)=w121, text=w108, error in=w69) -> (refnum out=w123:refnum<file>, error out=w124:errorcluster)  [unwired: 1 in, 1 out]
    n502 = Close File(refnum=w123, error in=w124) -> (error out=w67:errorcluster)  [unwired: 1 out]
    n503 = local write "Serial port data"(w127) -> ()
  }
  "error out" <- w27
  "Timings Indicator" <- w17
  "Is max" <- w11
  "Id max" <- w11
  "Ig max" <- w11
  "Imax vs time" <- w7
  "I vs Vg" <- w7
  "Imin vs time" <- w7
  "I vs Vd" <- w7
  "Serial port data" <- "" ("Serial port data")
  "Is min" <- w10
  "Id min" <- w10
  "Ig min" <- w10
  "Ion vs time" <- w7
  "Ioff vs time" <- w7
  "Is on" <- w9
  "Id on" <- w9
  "Ig on" <- w9
  "Is off" <- w8
  "Id off" <- w8
  "Ig off" <- w8
